vi "运维调试_总磷总氮.vi"() -> ()   [LabVIEW 2016, in "斯坦道氨氮.lvlib"]
uses:
  <vilib>/Utility/miscctls.llb/LVStringsAndValuesArrayTypeDef_U16.ctl
  <vilib>/Utility/miscctls.llb/LVPointTypeDef.ctl
  <vilib>/Plasmionique/MB Master/MB_Master/MB_Master.lvclass
  <vilib>/Utility/config.llb/NI_LVConfig.lvlib
  <vilib>/ptbypt/NI_PtbyPt.lvlib
panel:
  in  "灯值调整":bool
  in  "测试量程配置":T1
  in  "启动参数设置":bool
  out "固件版本号":string
  in  "定时设置":cluster{"启动":bool, "控制命令":T2, "测量参数":T3}(xcontrol)
  out "模块版本号":string
  out "温度2":sgl
  out "温度1":sgl
  out "ADC":sgl
  out "F3":sgl format="%#.6f"
  out "F2":sgl format="%#.6f"
  out "F1":sgl format="%#.6f"
  out "F0":sgl format="%#.6f"
  out "运行状态":T4 {"数据时间:" format="%<%y/%m/%d %H:%M:%S>T"; "仪器时间:" format="%<%y/%m/%d %H:%M:%S>T"}
  in  "单选按钮":enum32{"COD", "NH3N", "TN", "TP"}(radio)=enum."TN"
  in  "仪器参数":bool
  out "二级权限":bool
  out "一级权限":bool
  out "输入密码":u32
  out "布尔":bool
  in  "流程固件":bool
  in  "量程参数读取":T5
  in  "模块启用":bool
  in  "串口设置":bool
  in  "公式一键写入":bool
  in  "流程路径":path=path "data/流程.xml"
  in  "曲线模型":cluster{"X^2":dbl, "X":dbl, "B":dbl, "r^2":dbl}(xcontrol)
  out "字符串 2":string
  in  "质控参数设置":bool
  in  "数组":string[](array[string])
  in  "量程切换阈值写入":bool
  in  "量程切换阈值读取":bool
  in  "参数下拉列表":enum16{"COD", "氨氮", "总氮", "总磷"}(ring)
  in  "量程下拉列表":enum16{"低量程", "高量程"}(ring)
  in  "测量模式下拉列表":enum16{"水样测量", "零点核查", "跨度核查", "标样核查", "加标回收"}(ring)
  in  "公式":cluster{"X^2":dbl, "X":dbl, "b":dbl}
  in  "写公式":bool
  in  "读公式":bool
  in  "返回":bool
  in  "参数设置":bool
  out "集成报警信息":string
  in  "停止":bool
  in  "手动启动":bool
  in  "单步测试":bool
  out "多列列表框":i32(listbox)
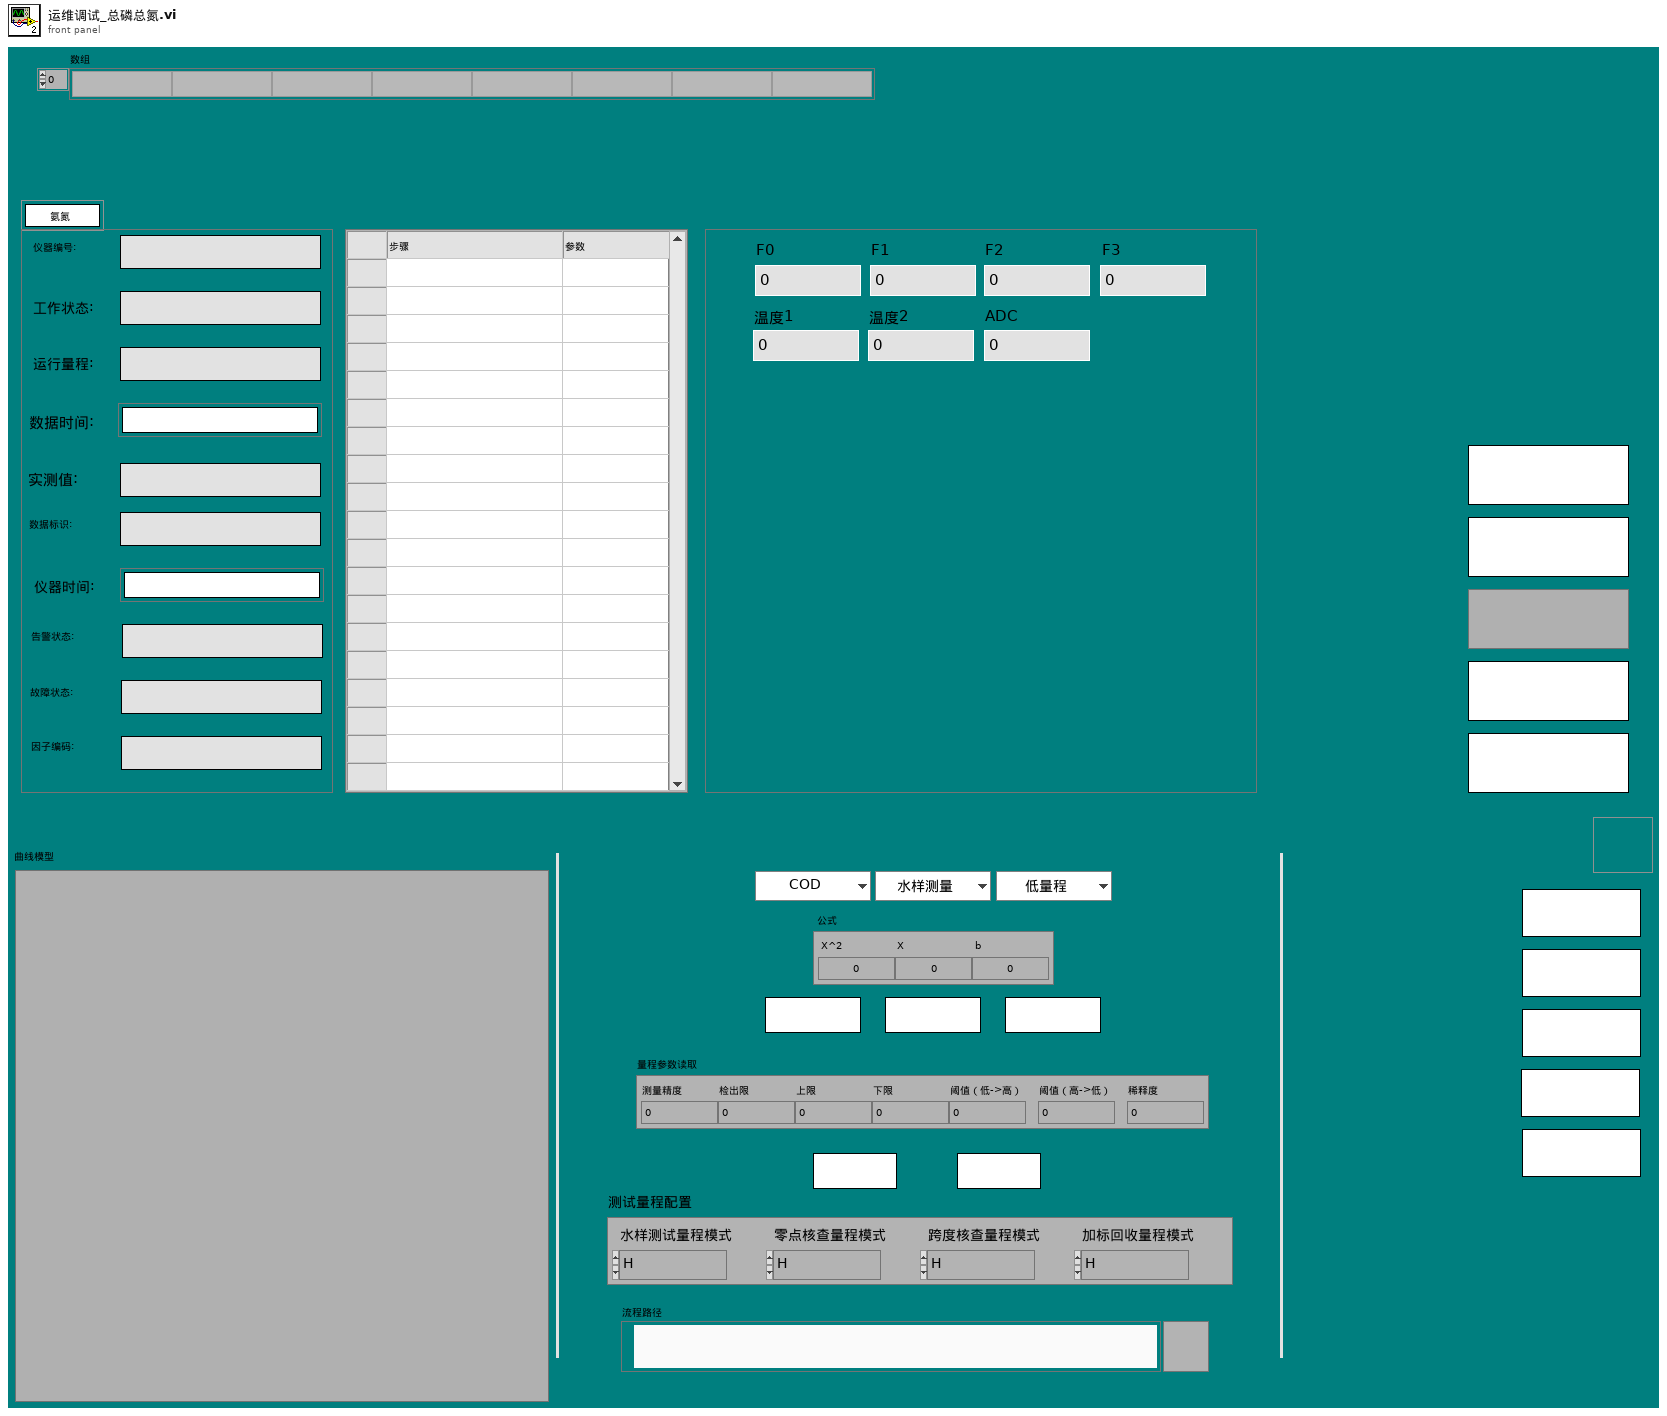
[diagram p1: front panel]
types:
  T1 = cluster{"水样测试量程模式":enum16{"H", "L", "AUTO"}, "空白核查量程模式":enum16{"H", "L", "AUTO"}, "跨度核查量程模式":enum16{"H", "L", "AUTO"}, "跨度核查量程模式 2":enum16{"H", "L", "AUTO"}}
  T2 = typedef "定时设置.xctl/国标控制命令.ctl" = enum16{"启动测量", "标样核查", "零点核查", "跨度核查", "空白测试", "平行样测试", "加标回收", "空白校准", "标样校准", "初始化（清洗）", "停止测试", "仪器重启", "校时", "模式设置", "测量间隔设置"}
  T3 = typedef "定时设置.xctl/测量参数.ctl" = u16
  T4 = cluster{"仪器编号:":string, "工作状态:":string, "运行量程: ":string, "数据时间:":timestamp, "实测值:":string, "数据标识: ":string, "仪器时间:":timestamp, "告警状态: ":string, "故障状态:  ":string, "因子编码:":string}
  T5 = cluster{"测量精度":dbl, "检出限":dbl, "上限":dbl, "下限":dbl, "阈值（低->高）":dbl, "阈值（高->低）":dbl, "稀释度":dbl}
  T6 = cluster{"时间源选择":enum16{"系统时间源", "仪器时间源"}, "外部时间源":timestamp}
  T7 = cluster{"系统时间":timestamp, "工作状态":enum16{"空闲", "水样测试", "标样核查", "零点核查", "跨度核查", "空白测试", "平行样测试", "加标回收", "空白校准", "标样校准", "初始化（清洗）"}, "测量模式":enum16{"待机", "连续模式", "周期模式", "定点模式", "受控模式", "手动模式"}, "告警代码":u16, "故障代码":u16, "日志代码":u16, "软件版本":u16, "F0":sgl, "F1":sgl, "F2":sgl, "F3":sgl, "T":sgl, "H":sgl, "id":u16, "flowid":u16, "量程":u16, "总磷控温温度1":sgl, "营养盐控温温度2":sgl, "ADC":sgl}
  T8 = enum32{"Bad", "Idle", "Run top level", "Running"}
  T9 = enum16{"空闲", "水样测试", "标样核查", "零点核查", "跨度核查", "空白测试", "平行样测试", "加标回收", "空白校准", "标样校准", "初始化（清洗）"}
  T10 = cluster{"水样测试量程模式":enum16{"H", "L", "AUTO"}, "空白核查量程模式":enum16{"H", "L", "AUTO"}, "跨度核查量程模式":enum16{"H", "L", "AUTO"}, "加标回收量程模式":enum16{"H", "L", "AUTO"}}
  T11 = typedef "LVStringsAndValuesArrayTypeDef_U16.ctl" = cluster{"String":string, "Value":u16}[]
  T12 = cluster{"COD":bool, "氨氮":bool, "总氮":bool, "总磷":bool}
  T13 = typedef "LVPointTypeDef.ctl" = cluster{"Horizontal":i16, "Vertical":i16}
  T14 = cluster{"因子编码":u32, "单位":u16, "标样参考值":sgl, "水样数据时间":timestamp, "水样实测值":sgl, "水样数据标识":string, "标样数据时间":timestamp, "标样实测值":sgl, "标样数据标识":string, "空白数据时间":timestamp, "空白实测值":sgl, "空白数据标识":string, "零点核查数据时间":timestamp, "零点核查实测值":sgl, "零点核查数据标识":string, "跨度核查数据时间":timestamp, "跨度核查实测值":sgl, "跨度核查数据标识":string, "加标回收数据时间":timestamp, "加标回收实测值":sgl, "加标回收数据标识":string, "平行样数据时间":timestamp, "平行样实测值":sgl, "平行样数据标识":string, "F0":sgl, "F1":sgl, "F2":sgl, "F3":sgl, "F4":sgl, "F5":sgl, "F6":sgl, "F7":sgl, "温度":sgl, "湿度":sgl, "X值":sgl, "fidrange":u16}
  T15 = cluster{"时间标识":timestamp, "设备":string, "日志信息":string, "备注":string}
  T16 = cluster{"参数":string, "报警内容":string, "报警分析":string}
  T17 = typedef "NI_LVConfig.lvlib/Config Data RefNum.ctl" = refnum<k1>
  T18 = cluster{"启动模式":enum16{"跨度核查", "水样测量", "空白核查", "标样核查", "加标回收"}, "启动参数":u16, "量程":enum16{"低量程", "高量程"}}
  T19 = cluster{"时间标识":timestamp, "设备":string, "日志信息":string, "流程参数":string}
  T20 = typedef "LVRowAndColumnUnsignedTypeDef.ctl" = cluster{"Row":u32, "Column":u32}
  T21 = cluster{"Major":u16, "Minor":u16, "Fix":u16, "Build":u16}
  T22 = cluster{"站号":u16, "量程切换":enum32{"H", "L", "AUTO"}, "控制命令":enum16{"启动测量", "标样核查", "零点核查", "跨度核查", "空白测试", "平行样测试", "加标回收", "空白校准", "标样校准", "初始化（清洗）", "停止测试", "仪器重启", "校时", "模式设置", "测量间隔设置"}, "模式设置":enum16{"待机", "连续模式", "周期模式", "定点模式", "受控模式", "手动模式"}, "测量间隔":u16}
  T23 = cluster{"参数下拉列表":enum16{"COD", "氨氮", "总氮", "总磷"}, "测量模式下拉列表":enum16{"水样测量", "零点核查", "跨度核查", "标样核查", "加标回收"}, "量程下拉列表":enum16{"低量程", "高量程"}}
  T24 = cluster{"被复制模型":cluster{"参数":u8, "测量模式":u8, "量程":u8}, "被覆盖模型":cluster{"参数":u8, "测量模式":u8, "量程":u8}[]}
  T25 = cluster{"总磷跨度值":dbl, "总磷零点标准液浓度":dbl, "总磷跨度标准液浓度":dbl, "总磷标准液标准浓度":dbl, "总氮跨度值":dbl, "总氮零点标准液浓度":dbl, "总氮跨度标准液浓度":dbl, "总氮标准液标准浓度":dbl, "COD跨度值":dbl, "COD零点标准液浓度":dbl, "COD跨度标准液浓度":dbl, "COD标准液标准浓度":dbl, "氨氮跨度值":dbl, "氨氮零点标准液浓度":dbl, "氨氮跨度标准液浓度":dbl, "氨氮标准液标准浓度":dbl}
  T26 = cluster{"测量量程":dbl, "测量精度":dbl, "测量间隔":dbl, "消解温度":dbl, "消解时长":dbl, "空白校准时间":timestamp, "曲线截距":dbl, "曲线斜率":dbl, "测量检出限":dbl, "测量信号值":dbl, "线性相关系数":dbl, "二次多项式系数":dbl, "标样校准时间":timestamp, "稀释倍数":dbl, "三项式系数":dbl, "空白标定系数":dbl, "量程系数":dbl, "F0/ORPA":dbl, "F1/ORPB":dbl, "F2/ORPK":dbl, "F3":dbl, "F4":dbl, "F5":dbl, "F6":dbl, "F7":dbl, "X0/滴定数":dbl, "量程":dbl}
  T27 = cluster{"COD仪器参数":cluster{"测量量程":dbl, "测量精度":dbl, "测量间隔":dbl, "消解温度":dbl, "消解时长":dbl, "空白校准时间":timestamp, "曲线截距":dbl, "曲线斜率":dbl, "测量检出限":dbl, "测量信号值":dbl, "线性相关系数":dbl, "二次多项式系数":dbl, "标样校准时间":timestamp, "稀释倍数":dbl, "三项式系数":dbl, "空白标定系数":dbl, "量程系数":dbl, "F0/ORPA":dbl, "F1/ORPB":dbl, "F2/ORPK":dbl, "F3":dbl, "F4":dbl, "F5":dbl, "F6":dbl, "F7":dbl, "X0/滴定数":dbl, "量程":dbl}, "氨氮仪器参数":cluster{"测量量程":dbl, "测量精度":dbl, "测量间隔":dbl, "消解温度":dbl, "消解时长":dbl, "空白校准时间":timestamp, "曲线截距":dbl, "曲线斜率":dbl, "测量检出限":dbl, "测量信号值":dbl, "线性相关系数":dbl, "二次多项式系数":dbl, "标样校准时间":timestamp, "稀释倍数":dbl, "三项式系数":dbl, "空白标定系数":dbl, "量程系数":dbl, "F0/ORPA":dbl, "F1/ORPB":dbl, "F2/ORPK":dbl, "F3":dbl, "F4":dbl, "F5":dbl, "F6":dbl, "F7":dbl, "X0/滴定数":dbl, "量程":dbl}, "总氮仪器参数":cluster{"测量量程":dbl, "测量精度":dbl, "测量间隔":dbl, "消解温度":dbl, "消解时长":dbl, "空白校准时间":timestamp, "曲线截距":dbl, "曲线斜率":dbl, "测量检出限":dbl, "测量信号值":dbl, "线性相关系数":dbl, "二次多项式系数":dbl, "标样校准时间":timestamp, "稀释倍数":dbl, "三项式系数":dbl, "空白标定系数":dbl, "量程系数":dbl, "F0/ORPA":dbl, "F1/ORPB":dbl, "F2/ORPK":dbl, "F3":dbl, "F4":dbl, "F5":dbl, "F6":dbl, "F7":dbl, "X0/滴定数":dbl, "量程":dbl}, "总磷仪器参数":cluster{"测量量程":dbl, "测量精度":dbl, "测量间隔":dbl, "消解温度":dbl, "消解时长":dbl, "空白校准时间":timestamp, "曲线截距":dbl, "曲线斜率":dbl, "测量检出限":dbl, "测量信号值":dbl, "线性相关系数":dbl, "二次多项式系数":dbl, "标样校准时间":timestamp, "稀释倍数":dbl, "三项式系数":dbl, "空白标定系数":dbl, "量程系数":dbl, "F0/ORPA":dbl, "F1/ORPB":dbl, "F2/ORPK":dbl, "F3":dbl, "F4":dbl, "F5":dbl, "F6":dbl, "F7":dbl, "X0/滴定数":dbl, "量程":dbl}}
  T28 = cluster{"测量精度":u16, "检出限":dbl, "上限":dbl, "下限":dbl, "阈值（低->高）":dbl, "阈值（高->低）":dbl, "稀释度":dbl}
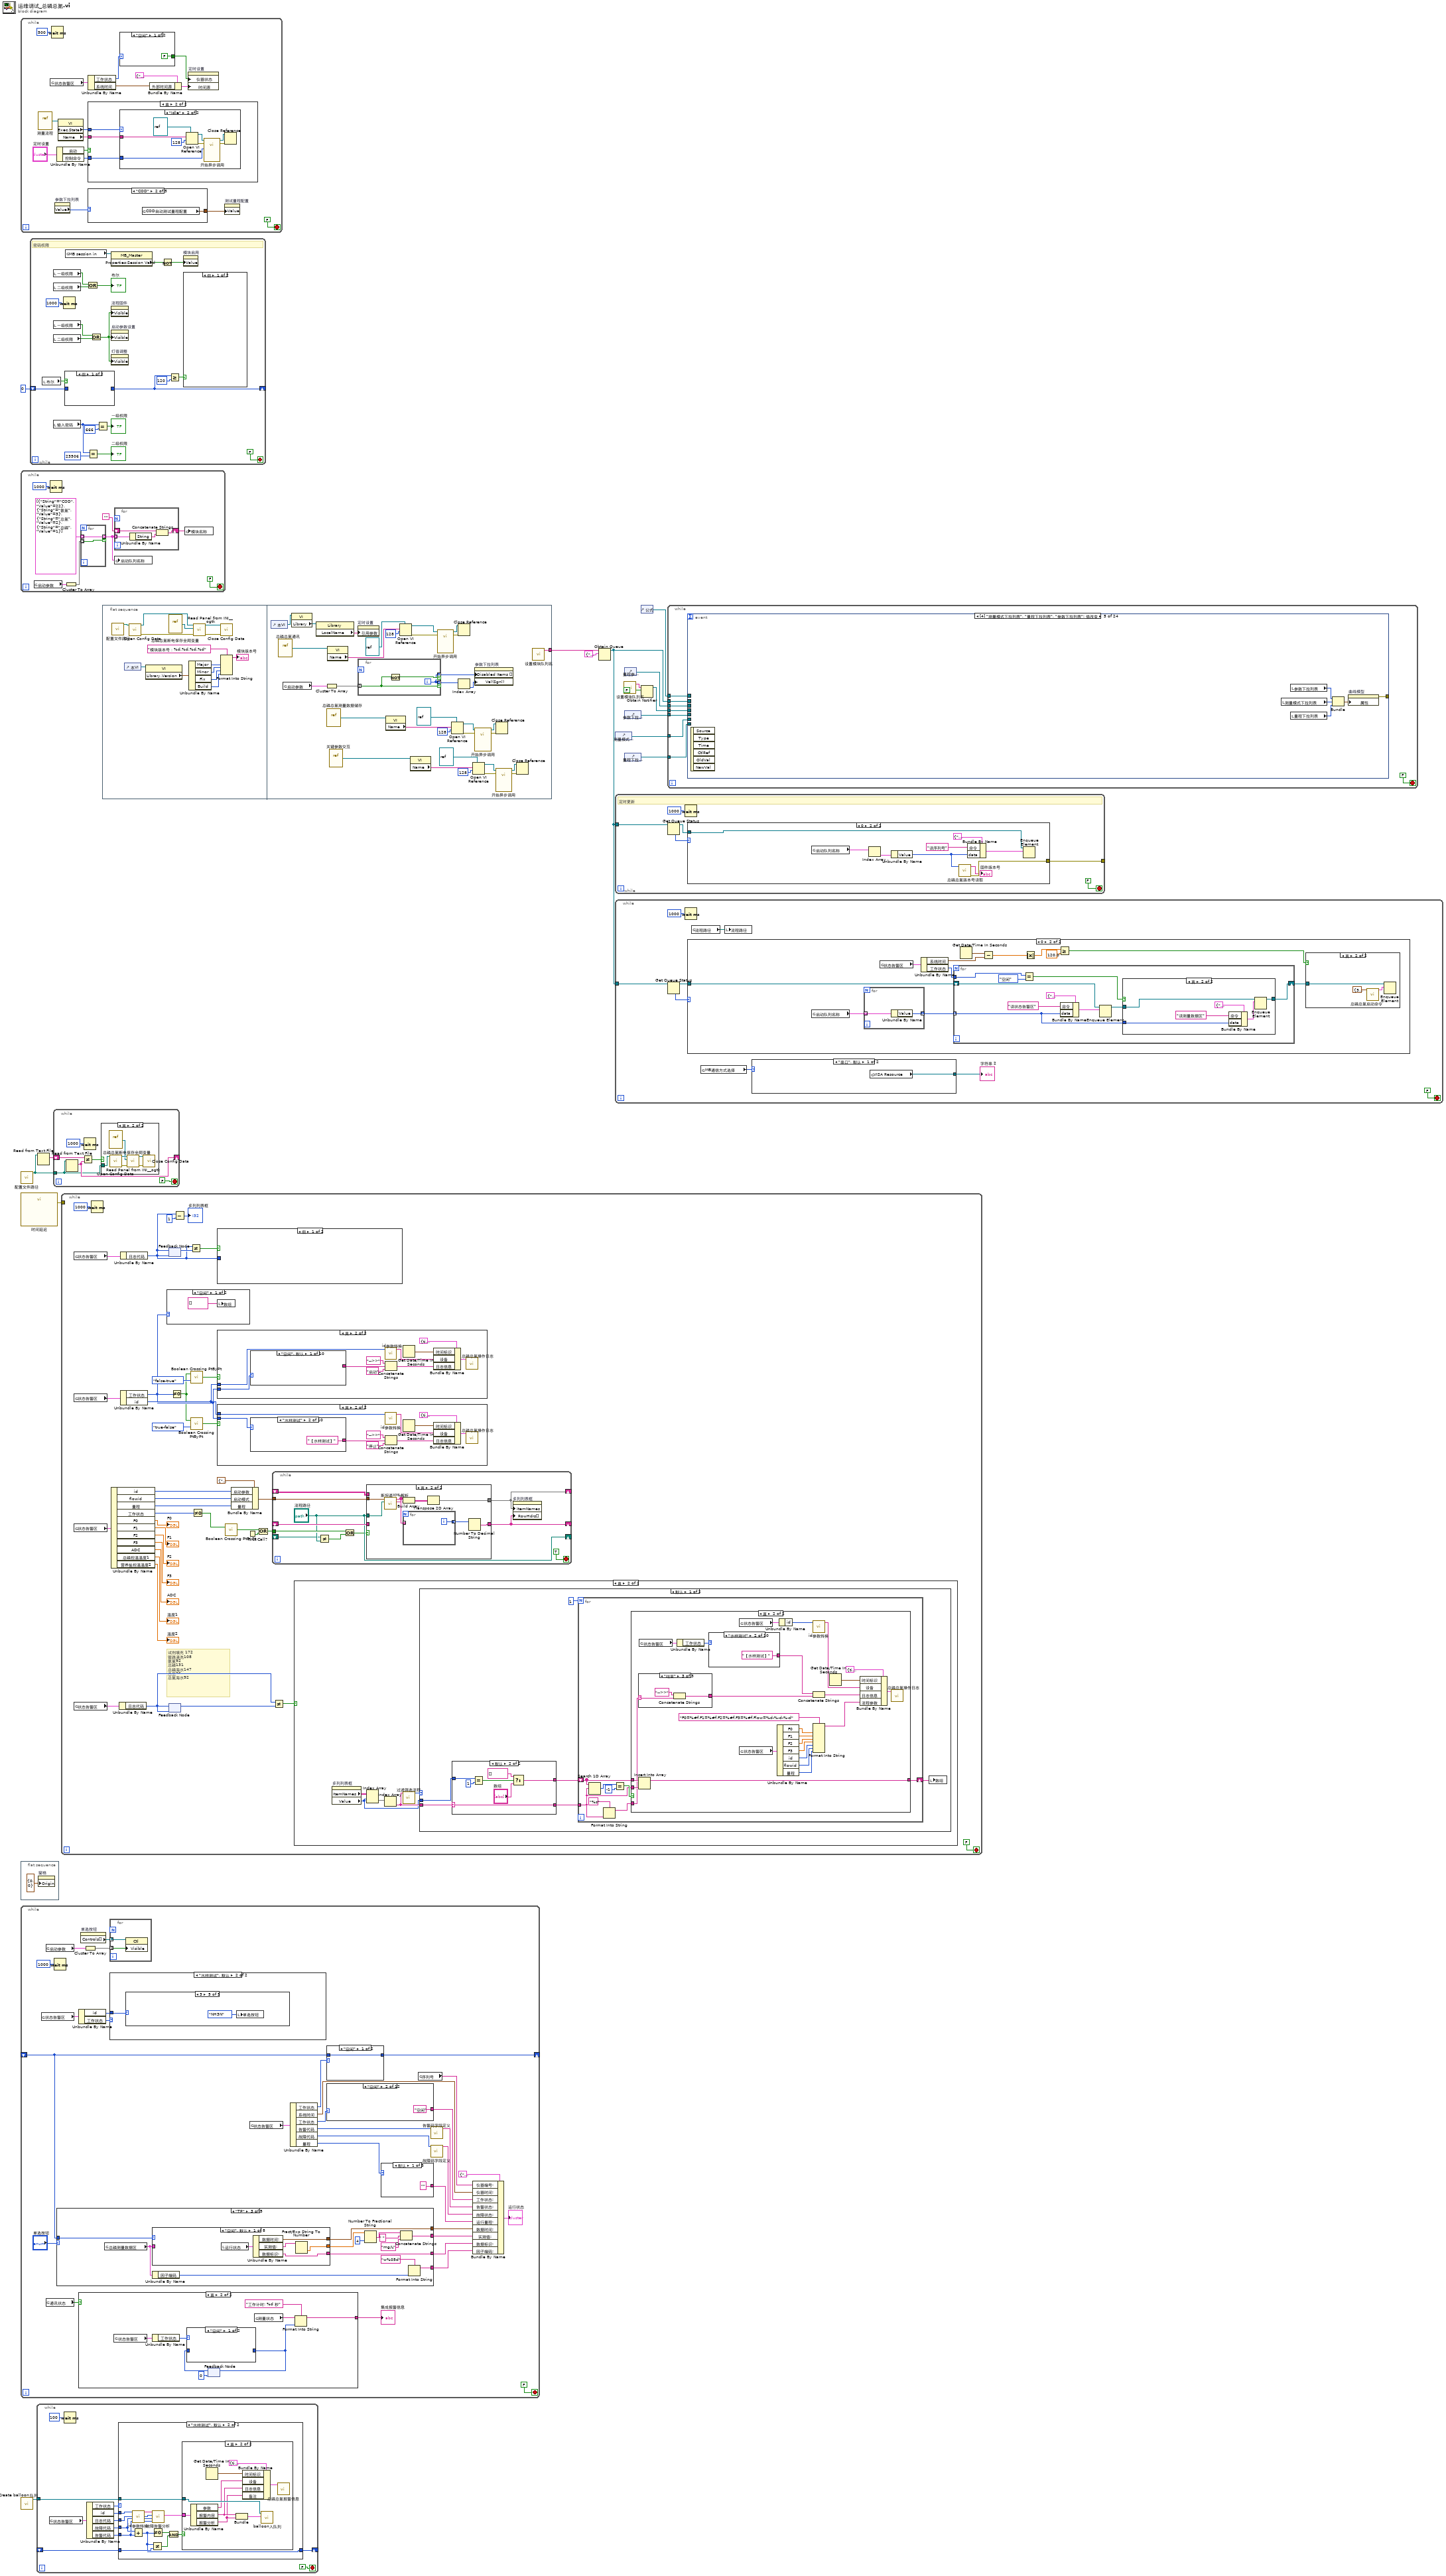
[diagram p0: block diagram]
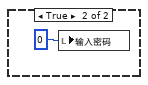
[diagram p5: hidden frame]
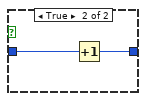
[diagram p6: hidden frame]
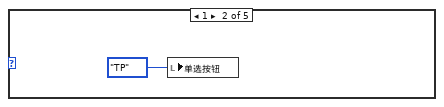
[diagram p11: hidden frame]
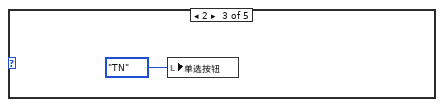
[diagram p12: hidden frame]
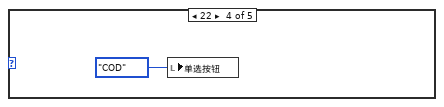
[diagram p13: hidden frame]
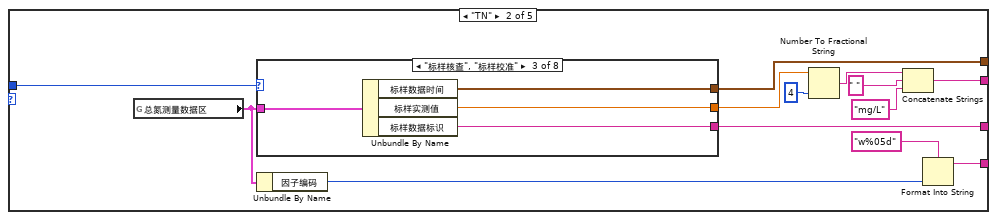
[diagram p15: hidden frame]
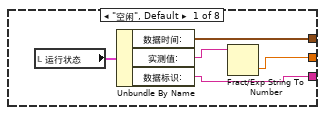
[diagram p16: hidden frame]
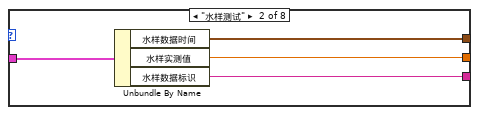
[diagram p17: hidden frame]
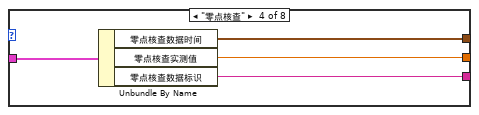
[diagram p18: hidden frame]
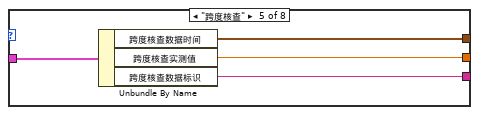
[diagram p19: hidden frame]
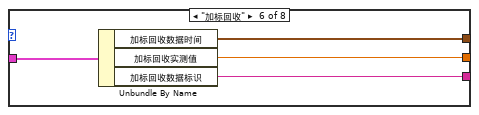
[diagram p20: hidden frame]
diagram:
  n1 = while {
    stop <- FALSE stop-if-true
    n2 = vi-ref "测量流程.vi"() -> (w30:refnum<vi>)
    n3 = global read "VAR总磷总氮全局变量.vi" "状态告警区"() -> (w27:T7)
    n4 = Wait (ms)(milliseconds to wait=u32 500 ("等待时间（毫秒）")) -> ()  [unwired: 1 out]
    n5 = property on="参数下拉列表" class="Enum (严格)"() -> ("Value"=w19:enum16{"COD", "氨氮", "总氮", "总磷"})  [unwired: 2 in, 2 out]
    n6 = Unbundle By Name("定时设置") -> ("启动"=w24:bool, "控制命令"=w23:T2)
    n7 = property class="VI"(reference=w30) -> ("Exec.State"=w29:T8, "Name"=w28:string)  [unwired: 1 in, 2 out]
    n8 = Unbundle By Name(w27) -> ("工作状态"=w26:T9, "系统时间"=w21:timestamp)
    n9 = case shown="真" w24 {
      tunnel: w28 -> [_ w41]
      tunnel: w23 -> [_ w40]
      tunnel: w29 -> [_ w39]
      frame False {
      }
      frame True {
        n10 = case shown="\"Idle\"" w39 {
          tunnel: w41 -> [_ w45]
          tunnel: w40 -> [_ w42]
          frame "Bad", Default {
          }
          frame "Idle" {
            n11 = Open VI Reference(type specifier VI Refnum (for type only)=refnum<vi> refnum, vi path=w45, options=128 ("选项")) -> (vi reference=w46:refnum<vi>, error out=w47:errorcluster)  [unwired: 3 in]
            n12 = call-by-ref "开始异步调用"(reference=w46, error in=w47, "控制命令"=w42) -> (reference out=w48:refnum<vi>, error out=w49:errorcluster)  [unwired: 11 in]
            n13 = Close Reference(reference=w48, error in (no error)=w49) -> ()  [unwired: 1 out]
          }
        }
      }
    }
    n14 = case shown="\"COD\"" w19 {
      tunnel: [_ w33 w34 w35 w36] -> w18
      frame Default {
      }
      frame "COD" {
        n15 = global read "总磷总氮断电保存全局变量.vi" "COD自动测试量程配置"() -> (w33:T10)
      }
      frame "氨氮" {
        n16 = global read "总磷总氮断电保存全局变量.vi" "氨氮自动测试量程配置"() -> (w34:T10)
      }
      frame "总氮" {
        n17 = global read "总磷总氮断电保存全局变量.vi" "总氮自动测试量程配置"() -> (w35:T10)
      }
      frame "总磷" {
        n18 = global read "总磷总氮断电保存全局变量.vi" "总磷自动测试量程配置"() -> (w36:T10)
      }
    }
    n19 = case shown="\"空闲\"" w26 {
      tunnel: [FALSE TRUE] -> w17
      frame "空闲" {
      }
      frame "水样测试", Default {
      }
    }
    n20 = Bundle By Name(cluster=T6 {"时间源选择"=enum."仪器时间源", "外部时间源"=timestamp(0 s since 1904-01-01)} ("时间源"), "外部时间源"=w21) -> (w20:T6)
    n21 = property on="定时设置" class="定时设置 (严格)"("仪器状态"=w17, "时间源"=w20) -> ()  [unwired: 2 in, 2 out]
    n22 = property on="测试量程配置" class="Clust (严格)"("Value"=w18) -> ()  [unwired: 2 in, 2 out]
  }
  n23 = while {
    stop <- FALSE stop-if-true
    n24 = global read "总磷总氮断电保存全局变量.vi" "启动参数"() -> (w55:T12)
    n25 = Wait (ms)(milliseconds to wait=u32 1000 ("等待时间（毫秒）")) -> ()  [unwired: 1 out]
    n26 = Cluster To Array(cluster=w55) -> (array=w54:bool[])
    n27 = for {
      tunnel: w54 -> [w63] mode=indexing
      tunnel: T11 [{"String"="COD", "Value"=22}, {"String"="氨氮", "Value"=3}, {"String"="总氮", "Value"=2}, {"String"="总磷", "Value"=1}] ("字符串与值[]") -> [w62] mode=indexing
      tunnel: [w62] -> w52 mode=indexing if=w63
    }
    n28 = for {
      tunnel: w52 -> [w61] mode=indexing
      shift-right: [w60] -> w50
      shift-left: "" -> [w58]
      n29 = Unbundle By Name(w61) -> ("String"=w59:string)
      n30 = Concatenate Strings(w58, w59) -> (w60:string)
    }
    n31 = global write "VAR总磷总氮全局变量.vi" "启动队列名称"(w52) -> ()
    n32 = global write "VAR总磷总氮全局变量.vi" "模块名称"(w50) -> ()
  }
  n33 = call "配置文件路径.vi"() -> ("appended path"=w4:path)  [unwired: 11 in]
  n34 = call "时间延迟"() -> ("error out"=w11:errorcluster)  [unwired: 11 in]
  n35 = flat-sequence {
    frame #0 {
      n36 = property on="窗格" class="Pane"("Origin"=T13 {"Horizontal"=0, "Vertical"=0} ("原点")) -> ()  [unwired: 2 in, 2 out]
    }
  }
  n37 = while {
    shift-right: [w66] -> _
    shift-left: _ -> [w65]
    stop <- FALSE stop-if-true
    n38 = global read "VAR总磷总氮全局变量.vi" "状态告警区"() -> (w77:T7)
    n39 = global read "总磷总氮断电保存全局变量.vi" "启动参数"() -> (w69:T12)
    n40 = global read "VAR总磷总氮全局变量.vi" "通讯状态"() -> (w93:bool)
    n41 = Wait (ms)(milliseconds to wait=u32 1000 ("等待时间（毫秒）")) -> ()  [unwired: 1 out]
    n42 = case shown="\"TP\"" "单选按钮" {
      tunnel: w65 -> [_ w109 w155 w201 w247]
      tunnel: [_ w108 w154 w199 w245] -> w81
      tunnel: [_ w107 w157 w203 w249] -> w80
      tunnel: [_ w106 w152 w197 w243] -> w79
      tunnel: [_ w105 w156 w202 w248] -> w78
      frame Default {
      }
      frame "TN" {
        n43 = global read "VAR总磷总氮全局变量.vi" "总氮测量数据区"() -> (w110:T14)
        n44 = case shown="\"标样核查\", \"标样校准\"" w109 {
          tunnel: [w120 w126 w130 w134 w138 w142 w146 w150] -> w108
          tunnel: [w118 w125 w129 w133 w136 w141 w145 w149] -> w112
          tunnel: [w121 w124 w128 w132 w135 w140 w144 w148] -> w106
          tunnel: w110 -> [_ w123 w127 w131 w137 w139 w143 w147]
          frame "空闲", Default {
            n45 = local read "运行状态"() -> (w122:T4)
            n46 = Unbundle By Name(w122) -> ("数据时间:"=w120:timestamp, "实测值:"=w119:string, "数据标识:"=w121:string)
            n47 = Fract/Exp String To Number(string=w119) -> (number=w118:dbl)  [unwired: 3 in, 1 out]
          }
          frame "水样测试" {
            n48 = Unbundle By Name(w123) -> ("水样数据时间"=w126:timestamp, "水样实测值"=w125:sgl, "水样数据标识"=w124:string)
          }
          frame "标样核查", "标样校准" {
            n49 = Unbundle By Name(w127) -> ("标样数据时间"=w130:timestamp, "标样实测值"=w129:sgl, "标样数据标识"=w128:string)
          }
          frame "零点核查" {
            n50 = Unbundle By Name(w131) -> ("零点核查数据时间"=w134:timestamp, "零点核查实测值"=w133:sgl, "零点核查数据标识"=w132:string)
          }
          frame "跨度核查" {
            n51 = Unbundle By Name(w137) -> ("跨度核查数据时间"=w138:timestamp, "跨度核查实测值"=w136:sgl, "跨度核查数据标识"=w135:string)
          }
          frame "加标回收" {
            n52 = Unbundle By Name(w139) -> ("加标回收数据时间"=w142:timestamp, "加标回收实测值"=w141:sgl, "加标回收数据标识"=w140:string)
          }
          frame "空白测试", "空白校准" {
            n53 = Unbundle By Name(w143) -> ("空白数据时间"=w146:timestamp, "空白实测值"=w145:sgl, "空白数据标识"=w144:string)
          }
          frame "平行样测试" {
            n54 = Unbundle By Name(w147) -> ("平行样数据时间"=w150:timestamp, "平行样实测值"=w149:sgl, "平行样数据标识"=w148:string)
          }
        }
        n55 = Unbundle By Name(w110) -> ("因子编码"=w116:u32)
        n56 = Number To Fractional String(number=w112, precision (6)=i16 4 ("精度(6)")) -> (F-format string=w114:string)  [unwired: 2 in]
        n57 = Concatenate Strings(w114, " " ("字符串"), "mg/L" ("字符串")) -> (w107:string)
        n58 = Format Into String(format string="w%05d" ("格式字符串"), w116) -> (resulting string=w105:string)  [unwired: 2 in, 1 out]
      }
      frame "TP" {
        n59 = global read "VAR总磷总氮全局变量.vi" "总磷测量数据区"() -> (w151:T14)
        n60 = case shown="\"空闲\", 默认" w155 {
          tunnel: [w166 w172 w176 w180 w184 w188 w192 w196] -> w154
          tunnel: [w164 w171 w175 w179 w182 w187 w191 w195] -> w153
          tunnel: [w167 w170 w174 w178 w181 w186 w190 w194] -> w152
          tunnel: w151 -> [_ w169 w173 w177 w183 w185 w189 w193]
          frame "空闲", Default {
            n61 = local read "运行状态"() -> (w168:T4)
            n62 = Unbundle By Name(w168) -> ("数据时间:"=w166:timestamp, "实测值:"=w165:string, "数据标识:"=w167:string)
            n63 = Fract/Exp String To Number(string=w165) -> (number=w164:dbl)  [unwired: 3 in, 1 out]
          }
          frame "水样测试" {
            n64 = Unbundle By Name(w169) -> ("水样数据时间"=w172:timestamp, "水样实测值"=w171:sgl, "水样数据标识"=w170:string)
          }
          frame "标样核查" {
            n65 = Unbundle By Name(w173) -> ("标样数据时间"=w176:timestamp, "标样实测值"=w175:sgl, "标样数据标识"=w174:string)
          }
          frame "零点核查" {
            n66 = Unbundle By Name(w177) -> ("零点核查数据时间"=w180:timestamp, "零点核查实测值"=w179:sgl, "零点核查数据标识"=w178:string)
          }
          frame "跨度核查" {
            n67 = Unbundle By Name(w183) -> ("跨度核查数据时间"=w184:timestamp, "跨度核查实测值"=w182:sgl, "跨度核查数据标识"=w181:string)
          }
          frame "加标回收" {
            n68 = Unbundle By Name(w185) -> ("加标回收数据时间"=w188:timestamp, "加标回收实测值"=w187:sgl, "加标回收数据标识"=w186:string)
          }
          frame "空白测试" {
            n69 = Unbundle By Name(w189) -> ("空白数据时间"=w192:timestamp, "空白实测值"=w191:sgl, "空白数据标识"=w190:string)
          }
          frame "平行样测试" {
            n70 = Unbundle By Name(w193) -> ("平行样数据时间"=w196:timestamp, "平行样实测值"=w195:sgl, "平行样数据标识"=w194:string)
          }
        }
        n71 = Unbundle By Name(w151) -> ("因子编码"=w162:u32)
        n72 = Number To Fractional String(number=w153, precision (6)=i16 4 ("精度(6)")) -> (F-format string=w160:string)  [unwired: 2 in]
        n73 = Concatenate Strings(w160, " " ("字符串"), "mg/L" ("字符串")) -> (w157:string)
        n74 = Format Into String(format string="w%05d" ("格式字符串"), w162) -> (resulting string=w156:string)  [unwired: 2 in, 1 out]
      }
      frame "NH3N" {
        n75 = global read "VAR总磷总氮全局变量.vi" "氨氮测量数据区"() -> (w200:T14)
        n76 = case shown="\"空闲\", 默认" w201 {
          tunnel: [w212 w218 w222 w226 w230 w234 w238 w242] -> w199
          tunnel: [w210 w217 w221 w225 w228 w233 w237 w241] -> w198
          tunnel: [w213 w216 w220 w224 w227 w232 w236 w240] -> w197
          tunnel: w200 -> [_ w215 w219 w223 w229 w231 w235 w239]
          frame "空闲", Default {
            n77 = local read "运行状态"() -> (w214:T4)
            n78 = Unbundle By Name(w214) -> ("数据时间:"=w212:timestamp, "实测值:"=w211:string, "数据标识:"=w213:string)
            n79 = Fract/Exp String To Number(string=w211) -> (number=w210:dbl)  [unwired: 3 in, 1 out]
          }
          frame "水样测试" {
            n80 = Unbundle By Name(w215) -> ("水样数据时间"=w218:timestamp, "水样实测值"=w217:sgl, "水样数据标识"=w216:string)
          }
          frame "标样核查" {
            n81 = Unbundle By Name(w219) -> ("标样数据时间"=w222:timestamp, "标样实测值"=w221:sgl, "标样数据标识"=w220:string)
          }
          frame "零点核查" {
            n82 = Unbundle By Name(w223) -> ("零点核查数据时间"=w226:timestamp, "零点核查实测值"=w225:sgl, "零点核查数据标识"=w224:string)
          }
          frame "跨度核查" {
            n83 = Unbundle By Name(w229) -> ("跨度核查数据时间"=w230:timestamp, "跨度核查实测值"=w228:sgl, "跨度核查数据标识"=w227:string)
          }
          frame "加标回收" {
            n84 = Unbundle By Name(w231) -> ("加标回收数据时间"=w234:timestamp, "加标回收实测值"=w233:sgl, "加标回收数据标识"=w232:string)
          }
          frame "空白测试" {
            n85 = Unbundle By Name(w235) -> ("空白数据时间"=w238:timestamp, "空白实测值"=w237:sgl, "空白数据标识"=w236:string)
          }
          frame "平行样测试" {
            n86 = Unbundle By Name(w239) -> ("平行样数据时间"=w242:timestamp, "平行样实测值"=w241:sgl, "平行样数据标识"=w240:string)
          }
        }
        n87 = Unbundle By Name(w200) -> ("因子编码"=w208:u32)
        n88 = Number To Fractional String(number=w198, precision (6)=i16 4 ("精度(6)")) -> (F-format string=w206:string)  [unwired: 2 in]
        n89 = Concatenate Strings(w206, " " ("字符串"), "mg/L" ("字符串")) -> (w203:string)
        n90 = Format Into String(format string="w%05d" ("格式字符串"), w208) -> (resulting string=w202:string)  [unwired: 2 in, 1 out]
      }
      frame "COD" {
        n91 = global read "VAR总磷总氮全局变量.vi" "COD测量数据区"() -> (w246:T14)
        n92 = case shown="\"空闲\", 默认" w247 {
          tunnel: [w258 w264 w268 w272 w276 w280 w284 w288] -> w245
          tunnel: [w256 w263 w267 w271 w274 w279 w283 w287] -> w244
          tunnel: [w259 w262 w266 w270 w273 w278 w282 w286] -> w243
          tunnel: w246 -> [_ w261 w265 w269 w275 w277 w281 w285]
          frame "空闲", Default {
            n93 = local read "运行状态"() -> (w260:T4)
            n94 = Unbundle By Name(w260) -> ("数据时间:"=w258:timestamp, "实测值:"=w257:string, "数据标识:"=w259:string)
            n95 = Fract/Exp String To Number(string=w257) -> (number=w256:dbl)  [unwired: 3 in, 1 out]
          }
          frame "水样测试" {
            n96 = Unbundle By Name(w261) -> ("水样数据时间"=w264:timestamp, "水样实测值"=w263:sgl, "水样数据标识"=w262:string)
          }
          frame "标样核查" {
            n97 = Unbundle By Name(w265) -> ("标样数据时间"=w268:timestamp, "标样实测值"=w267:sgl, "标样数据标识"=w266:string)
          }
          frame "零点核查" {
            n98 = Unbundle By Name(w269) -> ("零点核查数据时间"=w272:timestamp, "零点核查实测值"=w271:sgl, "零点核查数据标识"=w270:string)
          }
          frame "跨度核查" {
            n99 = Unbundle By Name(w275) -> ("跨度核查数据时间"=w276:timestamp, "跨度核查实测值"=w274:sgl, "跨度核查数据标识"=w273:string)
          }
          frame "加标回收" {
            n100 = Unbundle By Name(w277) -> ("加标回收数据时间"=w280:timestamp, "加标回收实测值"=w279:sgl, "加标回收数据标识"=w278:string)
          }
          frame "空白测试" {
            n101 = Unbundle By Name(w281) -> ("空白数据时间"=w284:timestamp, "空白实测值"=w283:sgl, "空白数据标识"=w282:string)
          }
          frame "平行样测试" {
            n102 = Unbundle By Name(w285) -> ("平行样数据时间"=w288:timestamp, "平行样实测值"=w287:sgl, "平行样数据标识"=w286:string)
          }
        }
        n103 = Unbundle By Name(w246) -> ("因子编码"=w254:u32)
        n104 = Number To Fractional String(number=w244, precision (6)=i16 4 ("精度(6)")) -> (F-format string=w252:string)  [unwired: 2 in]
        n105 = Concatenate Strings(w252, " " ("字符串"), "mg/L" ("字符串")) -> (w249:string)
        n106 = Format Into String(format string="w%05d" ("格式字符串"), w254) -> (resulting string=w248:string)  [unwired: 2 in, 1 out]
      }
    }
    n107 = Unbundle By Name(w77) -> ("id"=w76:u16, "工作状态"=w71:T9)
    n108 = case shown="真" w93 {
      tunnel: ["通讯异常" ("集成报警信息") w309] -> w92
      frame False {
      }
      frame True {
        n109 = global read "VAR总磷总氮全局变量.vi" "状态告警区"() -> (w315:T7)
        n110 = Unbundle By Name(w315) -> ("工作状态"=w314:T9)
        n111 = feedback #1(0) -> (w312:i32)
        n112 = case shown="\"空闲\"" w314 {
          tunnel: w312 -> [_ w317]
          tunnel: [_ w316] -> w310
          frame "空闲" {
          }
          frame Default {
            n113 = Increment(x=w317) -> (x+1=w316:i32)
          }
        }
        n114 = feedback-in #1(w310) -> ()
        n115 = global read "VAR总磷总氮全局变量.vi" "测量状态"() -> (w308:string)
        n116 = Format Into String(format string="工作计时: %d 秒" ("格式字符串"), initial string=w308, w310) -> (resulting string=w309:string)  [unwired: 1 in, 1 out]
      }
    }
    "集成报警信息" <- w92
    n117 = property on="单选按钮" class="RadioBtnsControl (严格)"() -> ("Controls[]"=w70:refnum<vi>[])  [unwired: 2 in, 2 out]
    n118 = Cluster To Array(cluster=w69) -> (array=w68:bool[])
    n119 = for {
      tunnel: w70 -> [w99] mode=indexing
      tunnel: w68 -> [w98] mode=indexing
      n120 = property class="Ctl"(reference=w99, "Visible"=w98) -> ()  [unwired: 1 in, 2 out]
    }
    n121 = case shown="\"水样测试\", 默认" w71 {
      tunnel: w76 -> [_ w100]
      frame "空闲" {
      }
      frame "水样测试", Default {
        n122 = case shown="3" w100 {
          frame 0, Default {
          }
          frame 1 {
            n123 = local write "单选按钮"(enum32{"COD", "NH3N", "TN", "TP"}."TP" ("单选按钮")) -> ()
          }
          frame 2 {
            n124 = local write "单选按钮"(enum32{"COD", "NH3N", "TN", "TP"}."TN" ("单选按钮")) -> ()
          }
          frame 22 {
            n125 = local write "单选按钮"(enum32{"COD", "NH3N", "TN", "TP"}."COD" ("单选按钮")) -> ()
          }
          frame 3 {
            n126 = local write "单选按钮"(enum32{"COD", "NH3N", "TN", "TP"}."NH3N" ("单选按钮")) -> ()
          }
        }
      }
    }
    n127 = global read "VAR总磷总氮全局变量.vi" "状态告警区"() -> (w91:T7)
    n128 = Unbundle By Name(w91) -> ("工作状态"=w67:T9, "系统时间"=w87:timestamp, "工作状态"=w86:T9, "告警代码"=w75:u16, "故障代码"=w73:u16, "量程"=w84:u16)
    n129 = case shown="\"空闲\"" w67 {
      selector: w67 -> [_ w97]
      tunnel: [w96 w97] -> w66
      tunnel: w65 -> [w96 _]
      frame "空闲" {
      }
      frame "水样测试", Default {
      }
    }
    n130 = case shown="\"空闲\"" w86 {
      selector: w86 -> [w292 _ _ _ _ _ _ _ _ _ _ _]
      tunnel: [w293 "空闲" ("工作状态") "水样测量" ("工作状态") "标样核查" ("工作状态") "零点核查" ("工作状态") "跨度核查" ("工作状态") "空白测试" ("工作状态") "平行样测试" ("工作状态") "加标回收" ("工作状态") "空白校准" ("工作状态") "标样校准" ("工作状态") "初始化" ("工作状态")] -> w85
      frame Default {
        n131 = Format Into String(format string="%d" ("格式字符串"), initial string="未知" ("工作状态"), w292) -> (resulting string=w293:string)  [unwired: 1 in, 1 out]
      }
      frame "空闲" {
      }
      frame "水样测试" {
      }
      frame "标样核查" {
      }
      frame "零点核查" {
      }
      frame "跨度核查" {
      }
      frame "空白测试" {
      }
      frame "平行样测试" {
      }
      frame "加标回收" {
      }
      frame "空白校准" {
      }
      frame "标样校准" {
      }
      frame "初始化（清洗）" {
      }
    }
    n132 = case shown="默认" w84 {
      tunnel: ["" ("字符串") "低量程" ("字符串") "高量程" ("字符串")] -> w83
      frame Default {
      }
      frame 0 {
      }
      frame 1 {
      }
    }
    n133 = global read "VAR总磷总氮全局变量.vi" "序列号"() -> (w88:string)
    n134 = call "告警码字段定义.vi"("告警代码"=w75) -> ("字符串"=w74:string)  [unwired: 8 in, 2 out]
    n135 = call "故障码字段定义.vi"("故障代码"=w73) -> ("字符串"=w72:string)  [unwired: 10 in]
    n136 = Bundle By Name(cluster=T4 {"仪器编号:"="", "工作状态:"="", "运行量程: "="", "数据时间:"=timestamp(0 s since 1904-01-01), "实测值:"="", "数据标识: "="", "仪器时间:"=timestamp(0 s since 1904-01-01), "告警状态: "="", "故障状态:  "="", "因子编码:"=""} ("运行状态"), "仪器编号:"=w88, "仪器时间:"=w87, "工作状态:"=w85, "告警状态:"=w74, "故障状态:"=w72, "运行量程:"=w83, "数据时间:"=w81, "实测值:"=w80, "数据标识:"=w79, "因子编码:"=w78) -> (→"运行状态":T4)
  }
  n137 = call "Create balloon 队列.vi"() -> ("队列输出"=w8:refnum<queue>)  [unwired: 11 in]
  n138 = while {
    shift-right: [w326] -> _
    shift-left: u32 0 ("y") -> [w328]
    stop <- FALSE stop-if-true
    # "密码权限"
    n139 = local read "布尔"() -> (w329:bool)
    n140 = local read "一级权限"() -> (w331:bool)
    n141 = local read "二级权限"() -> (w332:bool)
    n142 = local read "一级权限"() -> (w322:bool)
    n143 = local read "二级权限"() -> (w323:bool)
    n144 = local read "输入密码"() -> (w335:u32)
    n145 = Wait (ms)(milliseconds to wait=u32 1000 ("等待时间（毫秒）")) -> ()  [unwired: 1 out]
    n146 = case shown="假" w329 {
      tunnel: w328 -> [_ w341]
      tunnel: [_ w340] -> w326
      frame False {
      }
      frame True {
        n147 = Increment(x=w341) -> (x+1=w340:u32)
      }
    }
    n148 = global read "VAR总磷总氮全局变量.vi" "MB session in"() -> (w321:refnum<class "MB_Master.lvclass">)
    n149 = Or(x=w331, y=w332) -> (x .or. y?=→"布尔":bool)
    n150 = Equal?(x=w335, y=u32 23506) -> (x = y?=→"二级权限":bool)
    n151 = Or(x=w322, y=w323) -> (x .or. y?=w318:bool)
    n152 = Equal?(x=w335, y=u32 666) -> (x = y?=→"一级权限":bool)
    n153 = property class="MB_Master"(reference=w321) -> ("Properties:Session Valid"=w320:bool)  [unwired: 1 in, 2 out]
    n154 = property on="流程固件" class="Bool"("Visible"=w318) -> ()  [unwired: 2 in, 2 out]
    n155 = property on="启动参数设置" class="Bool"("Visible"=w318) -> ()  [unwired: 2 in, 2 out]
    n156 = property on="灯值调整" class="Bool"("Visible"=w318) -> ()  [unwired: 2 in, 2 out]
    n157 = Not(x=w320) -> (.not. x?=w319:bool)
    n158 = Greater Or Equal?(x=w326, y=u32 120) -> (x >= y?=w324:bool)
    n159 = property on="模块启用" class="Bool (严格)"("Value"=w319) -> ()  [unwired: 2 in, 2 out]
    n160 = case shown="假" w324 {
      frame False {
      }
      frame True {
        n161 = local write "输入密码"(u32 0 ("输入密码")) -> ()
      }
    }
  }
  n162 = while {
    tunnel: w8 -> [w348]
    shift-right: [w344] -> _
    shift-left: _ -> [w345]
    stop <- FALSE stop-if-true
    n163 = global read "VAR总磷总氮全局变量.vi" "状态告警区"() -> (w342:T7)
    n164 = Wait (ms)(milliseconds to wait=u32 100) -> ()  [unwired: 1 out]
    n165 = Unbundle By Name(w342) -> ("工作状态"=w343:T9, "id"=w350:u16, "日志代码"=w349:u16, "故障代码"=w347:u16, "告警代码"=w346:u16)
    n166 = case shown="\"水样测试\", 默认" w343 {
      tunnel: w350 -> [_ w365]
      tunnel: w349 -> [_ w364]
      tunnel: w348 -> [_ w361]
      tunnel: w347 -> [_ w360]
      tunnel: w346 -> [_ w359]
      tunnel: w345 -> [w353 w358]
      tunnel: [w353 w357] -> w344
      frame "空闲" {
      }
      frame "水样测试", Default {
        n167 = call "id参数转换.vi"("id"=w365) -> ("table输出"=w362:string)  [unwired: 10 in]
        n168 = Add(x=w360, y=w359) -> (x+y=w357:u16)
        n169 = Not Equal?(x=w357, y=w358) -> (x != y?=w355:bool)
        n170 = Not Equal To 0?(x=w357) -> (x != 0?=w356:bool)
        n171 = call "故障告警分析.vi"("告警代码"=w359, "故障代码"=w360, "运行步序"=w364, "参数"=w362) -> ("报警内容"=w363:T16)  [unwired: 6 in, 1 out]
        n172 = And(x=w356, y=w355) -> (x .and. y?=w354:bool)
        n173 = case shown="真" w354 {
          tunnel: w363 -> [_ w374]
          tunnel: w361 -> [_ w373]
          frame False {
          }
          frame True {
            n174 = Unbundle By Name(w374) -> ("参数"=w369:string, "报警内容"=w368:string, "报警分析"=w367:string)
            n175 = Get Date/Time In Seconds() -> (seconds since 1Jan1904=w372:timestamp)
            n176 = Bundle("报警内容"=w368, "报警分析"=w367) -> (w366:cluster{"报警内容":string, "报警分析":string})  [unwired: 1 in]
            n177 = Bundle By Name(cluster=T15 {"时间标识"=timestamp(0 s since 1904-01-01), "设备"="", "日志信息"="", "备注"=""} ("data in"), "时间标识"=w372, "设备"=w369, "日志信息"=w368, "备注"=w367) -> (w371:T15)
            n178 = call "balloon入队列.vi"("报警内容"=w366, "队列"=w373) -> ()  [unwired: 9 in, 1 out]
            n179 = call "总磷总氮报警信息.vi"("data in"=w371) -> ()  [unwired: 10 in, 1 out]
          }
        }
      }
    }
  }
  n180 = Read from Text File(file (use dialog)=w4) -> (text=w5:string)  [unwired: 3 in, 3 out]
  n181 = while {
    shift-right: [w377] -> _
    shift-left: w5 -> [w379]
    tunnel: w4 -> [w376]
    stop <- FALSE stop-if-true
    n182 = Read from Text File(file (use dialog)=w376) -> (text=w377:string)  [unwired: 3 in, 3 out]
    n183 = Not Equal?(x=w379, y=w377) -> (x != y?=w378:bool)
    n184 = Wait (ms)(milliseconds to wait=u32 1000 ("等待时间（毫秒）")) -> ()  [unwired: 1 out]
    n185 = case shown="真" w378 {
      tunnel: w376 -> [_ w381]
      frame False {
      }
      frame True {
        n186 = vi-ref "总磷总氮断电保存全局变量.vi"() -> (w385:refnum<vi>)
        n187 = call <vilib>:"Open Config Data.vi"("configuration file path"=w381) -> ("error out"=w383:errorcluster, "refnum"=w386:T17)  [unwired: 8 in, 1 out]
        n188 = call <userlib>:"Read Panel from INI__ogtk.vi"("error in (no error)"=w383, "VI ref"=w385, "refnum"=w386) -> ("error out"=w382:errorcluster, "refnum out"=w384:T17)  [unwired: 7 in]
        n189 = call <vilib>:"Close Config Data.vi"("error in (no error)"=w382, "refnum"=w384) -> ()  [unwired: 8 in, 2 out]
      }
    }
  }
  n190 = while {
    tunnel: w11 -> [_]
    stop <- FALSE stop-if-true
    # "试剂填充 172 \n管路清洗108\n氨氮92\n总磷131\n总磷海水147\n总氮76\n总氮海水92"
    n191 = global read "VAR总磷总氮全局变量.vi" "状态告警区"() -> (w413:T7)
    n192 = global read "VAR总磷总氮全局变量.vi" "状态告警区"() -> (w411:T7)
    n193 = global read "VAR总磷总氮全局变量.vi" "状态告警区"() -> (w417:T7)
    n194 = global read "VAR总磷总氮全局变量.vi" "状态告警区"() -> (w409:T7)
    n195 = Wait (ms)(milliseconds to wait=u32 1000 ("等待时间（毫秒）")) -> ()  [unwired: 1 out]
    n196 = Unbundle By Name(w417) -> ("id"=w414:u16, "flowid"=w416:u16, "量程"=w415:u16, "工作状态"=w402:T9, "F0"=→"F0":sgl, "F1"=→"F1":sgl, "F2"=→"F2":sgl, "F3"=→"F3":sgl, "ADC"=→"ADC":sgl, "总磷控温温度1"=→"温度1":sgl, "营养盐控温温度2"=→"温度2":sgl)
    n197 = Unbundle By Name(w409) -> ("日志代码"=w408:u16)
    n198 = Unbundle By Name(w413) -> ("日志代码"=w405:u16)
    n199 = Unbundle By Name(w411) -> ("工作状态"=w397:T9, "id"=w398:u16)
    n200 = case shown="\"空闲\"" w397 {
      frame "空闲" {
        n201 = local write "数组"(string[] [] ("数组")) -> ()
      }
      frame "水样测试", Default {
      }
    }
    n202 = feedback-in #2(w405) -> ()
    n203 = feedback #2(w405) -> (w422:u16)
    n204 = feedback #3(w408) -> (w410:u16)
    n205 = feedback-in #3(w408) -> ()
    n206 = Not Equal To 0?(x=w397) -> (x != 0?=w395:bool)
    n207 = Subtract(x=w405, y=1) -> (x-y=→"多列列表框":i32)
    n208 = Not Equal?(x=w405, y=w422) -> (x != y?=w421:bool)
    n209 = call <vilib>:"Boolean Crossing PtByPt.vi"("direction"=enum16{"either", "false-true", "true-false"}."false-true", "input"=w395) -> ("crossing"=w399:bool)  [unwired: 1 in]
    n210 = call <vilib>:"Boolean Crossing PtByPt.vi"("direction"=enum16{"either", "false-true", "true-false"}."true-false", "input"=w395) -> ("crossing"=w394:bool)  [unwired: 1 in]
    n211 = Not Equal To 0?(x=w402) -> (x != 0?=w419:bool)
    n212 = case shown="假" w421 {
      tunnel: w405 -> [_ w558]
      frame False {
      }
      frame True {
        n213 = Subtract(x=w558, y=1) -> (x-y=w556:i32)
        n214 = Subtract(x=w556, y=5) -> (x-y=w560:i32)
        n215 = Greater Or Equal To 0?(x=w560) -> (x >= 0?=w559:bool)
        n216 = property on="多列列表框" class="MCListbox (严格)"() -> (error out=w564:errorcluster, "TopLeft"=w565:T20)  [unwired: 2 in, 1 out]
        n217 = Select(t=w560, s=w559, f=0) -> (s? t:f=w561:i32)
        n218 = Bundle By Name(cluster=w565, "Row"=w561) -> (w566:T20)
        n219 = property on="多列列表框" class="MCListbox (严格)"(error in=w564, "TopLeft"=w566) -> ()  [unwired: 1 in, 2 out]
      }
    }
    n220 = case shown="真" w399 {
      tunnel: w397 -> [_ w448]
      tunnel: w398 -> [_ w445]
      frame False {
      }
      frame True {
        n221 = case shown="\"空闲\", 默认" w448 {
          tunnel: [_ "【水样测试】" ("字符串") "【标样核查】" ("字符串") "【零点核查】" ("字符串") "【跨度核查】" ("字符串") "【空白测试】" ("字符串") "【平行样测试】" ("字符串") "【加标回收】" ("字符串") "【空白校准】" ("字符串") "【标样校准】" ("字符串")] -> w453
          frame "空闲", Default {
          }
          frame "水样测试" {
          }
          frame "标样核查" {
          }
          frame "零点核查" {
          }
          frame "跨度核查" {
          }
          frame "空白测试" {
          }
          frame "平行样测试" {
          }
          frame "加标回收" {
          }
          frame "空白校准" {
          }
          frame "标样校准" {
          }
        }
        n222 = call "id参数转换.vi"("id"=w445) -> ("table输出"=w444:string)  [unwired: 10 in]
        n223 = Concatenate Strings("-->>" ("字符串"), w453, "启动" ("字符串")) -> (w452:string)
        n224 = Get Date/Time In Seconds() -> (seconds since 1Jan1904=w450:timestamp)
        n225 = Bundle By Name(cluster=T19 {"时间标识"=timestamp(0 s since 1904-01-01), "设备"="", "日志信息"="", "流程参数"=""} ("data in"), "时间标识"=w450, "设备"=w444, "日志信息"=w452) -> (w449:T19)
        n226 = call "总磷总氮操作日志.vi"("data in"=w449) -> ()  [unwired: 11 in]
      }
    }
    n227 = case shown="真" w394 {
      tunnel: w397 -> [_ w429]
      tunnel: w398 -> [_ w426]
      frame False {
      }
      frame True {
        n228 = case shown="\"水样测试\"" w429 {
          tunnel: [_ "【水样测试】" ("字符串") "【标样核查】" ("字符串") "【零点核查】" ("字符串") "【跨度核查】" ("字符串") "【空白测试】" ("字符串") "【平行样测试】" ("字符串") "【加标回收】" ("字符串") "【空白校准】" ("字符串") "【标样校准】" ("字符串")] -> w434
          frame "空闲", Default {
          }
          frame "水样测试" {
          }
          frame "标样核查" {
          }
          frame "零点核查" {
          }
          frame "跨度核查" {
          }
          frame "空白测试" {
          }
          frame "平行样测试" {
          }
          frame "加标回收" {
          }
          frame "空白校准" {
          }
          frame "标样校准" {
          }
        }
        n229 = call "id参数转换.vi"("id"=w426) -> ("table输出"=w425:string)  [unwired: 10 in]
        n230 = Concatenate Strings("-->>" ("字符串"), w434, "停止" ("字符串")) -> (w433:string)
        n231 = Get Date/Time In Seconds() -> (seconds since 1Jan1904=w431:timestamp)
        n232 = Bundle By Name(cluster=T19 {"时间标识"=timestamp(0 s since 1904-01-01), "设备"="", "日志信息"="", "流程参数"=""} ("data in"), "时间标识"=w431, "设备"=w425, "日志信息"=w433) -> (w430:T19)
        n233 = call "总磷总氮操作日志.vi"("data in"=w430) -> ()  [unwired: 11 in]
      }
    }
    n234 = call <vilib>:"Boolean Crossing PtByPt.vi"("input"=w419) -> ("crossing"=w401:bool)  [unwired: 2 in]
    n235 = Bundle By Name(cluster=T18 {"启动模式"=enum."跨度核查", "启动参数"=1, "量程"=enum."低量程"} ("参数簇"), "启动参数"=w414, "启动模式"=w416, "量程"=w415) -> (w412:T18)
    n236 = First Call?() -> (First Call?: T/F=w420:bool)
    n237 = Or(x=w401, y=w420) -> (x .or. y?=w418:bool)
    n238 = while {
      tunnel: w418 -> [w544]
      tunnel: w412 -> [w543]
      shift-right: [w538] -> _
      shift-left: _ -> [w540]
      shift-right: [w539] -> _
      shift-left: _ -> [w541]
      shift-right: ["流程路径"] -> _
      shift-left: _ -> [w536]
      stop <- TRUE stop-if-true
      n239 = Not Equal?(x=w536, y="流程路径") -> (x != y?=w534:bool)
      n240 = Or(x=w544, y=w534) -> (x .or. y?=w535:bool)
      n241 = case shown="真" w535 {
        tunnel: [w546 w554] -> w539
        tunnel: [w545 w553] -> w538
        tunnel: w543 -> [_ w548]
        tunnel: w541 -> [w546 _]
        tunnel: w540 -> [w545 _]
        tunnel: "流程路径" -> [_ w547]
        frame False {
        }
        frame True {
          n242 = call "斯坦道XML解析.vi"("添加的路径"=w547, "参数簇"=w548) -> ("步骤时间"=w549:string[], "步骤名"=w551:string[])  [unwired: 8 in]
          n243 = Build Array(w551, w549) -> (w550:string[][])
          n244 = for {
            tunnel: w551 -> [_] mode=indexing
            tunnel: [w555] -> w552 mode=indexing
            i -> [w555]
          }
          n245 = Transpose 2D Array(2D array=w550) -> (transposed array=w553:string[][])
          n246 = Number To Decimal String(number=w552) -> (decimal integer string=w554:string[])  [unwired: 1 in]
        }
      }
      n247 = property on="多列列表框" class="MCListbox (严格)"("ItemNames"=w538, "RowHdrs[]"=w539) -> ()  [unwired: 2 in, 2 out]
    }
    n248 = Not Equal?(x=w408, y=w410) -> (x != y?=w407:bool)
    n249 = case shown="真" w407 {
      frame False {
      }
      frame True {
        n250 = property on="多列列表框" class="MCListbox (严格)"() -> ("ItemNames"=w468:string[][], "Value"=w464:i32)  [unwired: 2 in, 2 out]
        n251 = Index Array(array=w468, index (row)=w464) -> (element=w467:string[])  [unwired: 1 in]
        n252 = Index Array(array=w467) -> (element=w466:string)  [unwired: 1 in]
        n253 = call "过滤筛选流程.vi"("字符串"=w466) -> ("匹配后偏移量"=w465:i32)  [unwired: 10 in]
        n254 = case shown="默认" w465 {
          tunnel: w466 -> [w470 _]
          tunnel: w464 -> [w469 _]
          frame Default {
            n255 = case shown="默认" w470 {
              selector: w470 -> [w476 w483]
              tunnel: [w476 w483] -> w472
              tunnel: [string[] [] ("数组") w478] -> w471
              tunnel: w469 -> [_ w482]
              frame "读数" {
              }
              frame Default {
                n256 = Equal?(x=w482, y=1) -> (x = y?=w480:bool)
                n257 = Select(t=string[] [], s=w480, f="数组") -> (s? t:f=w478:string[])
              }
            }
            n258 = for {
              N: 1 -> [_]
              tunnel: w472 -> [w485]
              shift-right: [w484] -> w473
              shift-left: w471 -> [w486]
              n259 = Search 1D Array(1D array=w486, element=w485) -> (index of element=w489:i32)  [unwired: 1 in]
              n260 = Format Into String(format string="%s" ("格式字符串"), w485) -> (resulting string=w490:string)  [unwired: 2 in, 1 out]
              n261 = Equal?(x=w489, y=-1) -> (x = y?=w487:bool)
              n262 = case shown="真" w487 {
                tunnel: w490 -> [_ w500]
                tunnel: w486 -> [w492 w504]
                tunnel: w485 -> [_ w503]
                tunnel: [w492 w502] -> w484
                frame False {
                }
                frame True {
                  n263 = case shown="\"结束\"" w500 {
                    selector: w500 -> [w527 w530 w533]
                    tunnel: [w527 w529 w532] -> w499
                    frame Default {
                    }
                    frame "初始化" {
                      n264 = Concatenate Strings("-->>" ("字符串"), w530) -> (w529:string)
                    }
                    frame "结束" {
                      n265 = Concatenate Strings("-->>" ("字符串"), w533) -> (w532:string)
                    }
                  }
                  n266 = Insert Into Array(array=w504, new element=w503) -> (w502:string[])  [unwired: 1 in]
                  n267 = global read "VAR总磷总氮全局变量.vi" "状态告警区"() -> (w498:T7)
                  n268 = Unbundle By Name(w498) -> ("工作状态"=w497:T9)
                  n269 = case shown="\"水样测试\"" w497 {
                    tunnel: [_ "【水样测试】" ("字符串") "【标样核查】" ("字符串") "【零点核查】" ("字符串") "【跨度核查】" ("字符串") "【空白测试】" ("字符串") "【平行样测试】" ("字符串") "【加标回收】" ("字符串") "【空白校准】" ("字符串") "【标样校准】" ("字符串")] -> w495
                    frame "空闲", Default {
                    }
                    frame "水样测试" {
                    }
                    frame "标样核查" {
                    }
                    frame "零点核查" {
                    }
                    frame "跨度核查" {
                    }
                    frame "空白测试" {
                    }
                    frame "平行样测试" {
                    }
                    frame "加标回收" {
                    }
                    frame "空白校准" {
                    }
                    frame "标样校准" {
                    }
                  }
                  n270 = global read "VAR总磷总氮全局变量.vi" "状态告警区"() -> (w517:T7)
                  n271 = global read "VAR总磷总氮全局变量.vi" "状态告警区"() -> (w514:T7)
                  n272 = Unbundle By Name(w514) -> ("F0"=w511:sgl, "F1"=w510:sgl, "F2"=w509:sgl, "F3"=w508:sgl, "id"=w507:u16, "flowid"=w506:u16, "量程"=w505:u16)
                  n273 = Unbundle By Name(w517) -> ("id"=w494:u16)
                  n274 = call "id参数转换.vi"("id"=w494) -> ("table输出"=w493:string)  [unwired: 10 in]
                  n275 = Concatenate Strings(w495, w499) -> (w496:string)
                  n276 = Format Into String(format string="F0=%#f,F1=%#f,F2=%#f,F3=%#f,Flow=%d-%-d-%-d" ("格式字符串"), w511, w510, w509, w508, w507, w506, w505) -> (resulting string=w512:string)  [unwired: 2 in, 1 out]
                  n277 = Get Date/Time In Seconds() -> (seconds since 1Jan1904=w515:timestamp)
                  n278 = Bundle By Name(cluster=T19 {"时间标识"=timestamp(0 s since 1904-01-01), "设备"="", "日志信息"="", "流程参数"=""} ("data in"), "时间标识"=w515, "设备"=w493, "日志信息"=w496, "流程参数"=w512) -> (w516:T19)
                  n279 = call "总磷总氮操作日志.vi"("data in"=w516) -> ()  [unwired: 11 in]
                }
              }
            }
            n280 = local write "数组"(w473) -> ()
          }
          frame -1 {
          }
        }
      }
    }
  }
  n281 = flat-sequence {
    tunnel: [w582] -> w6
    frame #0 {
      n282 = call "配置文件路径.vi"() -> ("appended path"=w575:path)  [unwired: 11 in]
      n283 = control-ref of="本VI"() -> (w574:refnum<vi>)
      n284 = call <vilib>:"Open Config Data.vi"("configuration file path"=w575) -> ("error out"=w579:errorcluster, "refnum"=w576:T17)  [unwired: 8 in, 1 out]
      n285 = property class="VI"(reference=w574) -> ("Library.Version"=w573:T21)  [unwired: 1 in, 2 out]
      n286 = vi-ref "总磷总氮断电保存全局变量.vi"() -> (w577:refnum<vi>)
      n287 = Unbundle By Name(w573) -> ("Major"=w571:u16, "Minor"=w570:u16, "Fix"=w569:u16, "Build"=w568:u16)
      n288 = call <userlib>:"Read Panel from INI__ogtk.vi"("error in (no error)"=w579, "VI ref"=w577, "refnum"=w576) -> ("error out"=w580:errorcluster, "refnum out"=w578:T17)  [unwired: 7 in]
      n289 = call <vilib>:"Close Config Data.vi"("error in (no error)"=w580, "refnum"=w578) -> ()  [unwired: 8 in, 2 out]
      n290 = Format Into String(format string="模块版本号：%d.%d.%d.%d" ("格式字符串"), w571, w570, w569, w568) -> (resulting string=→"模块版本号":string)  [unwired: 2 in, 1 out]
    }
    frame #1 {
      n291 = control-ref of="本VI"() -> (w583:refnum<vi>)
      n292 = vi-ref "总磷总氮通讯.vi"() -> (w598:refnum<vi>)
      n293 = global read "总磷总氮断电保存全局变量.vi" "启动参数"() -> (w586:T12)
      n294 = property class="VI"(reference=w583) -> ("Library"=w584:refnum<vi>)  [unwired: 1 in, 2 out]
      n295 = property class="Library"(reference=w584) -> ("LocalName"=w585:string)  [unwired: 1 in, 2 out]
      n296 = Cluster To Array(cluster=w586) -> (array=w587:bool[])
      n297 = vi-ref "总磷总氮测量数据储存.vi"() -> (w606:refnum<vi>)
      n298 = property class="VI"(reference=w598) -> ("Name"=w599:string)  [unwired: 1 in, 2 out]
      n299 = vi-ref "关键参数交互.vi"() -> (w597:refnum<vi>)
      n300 = property on="定时设置" class="定时设置 (严格)"("引用参数"=w585) -> ()  [unwired: 2 in, 2 out]
      n301 = for {
        tunnel: w587 -> [w614] mode=indexing
        tunnel: [w615] -> w589 mode=indexing if=w616
        tunnel: [w615] -> w588 mode=indexing if=w614
        i -> [w615]
        n302 = Not(x=w614) -> (.not. x?=w616:bool)
      }
      n303 = property class="VI"(reference=w606) -> ("Name"=w613:string)  [unwired: 1 in, 2 out]
      n304 = Open VI Reference(type specifier VI Refnum (for type only)=refnum<vi> refnum, vi path=w599, options=128 ("选项")) -> (vi reference=w601:refnum<vi>, error out=w603:errorcluster)  [unwired: 3 in]
      n305 = property class="VI"(reference=w597) -> ("Name"=w591:string)  [unwired: 1 in, 2 out]
      n306 = call-by-ref "开始异步调用"(reference=w601, error in=w603) -> (reference out=w605:refnum<vi>, error out=w604:errorcluster)  [unwired: 12 in]
      n307 = Open VI Reference(type specifier VI Refnum (for type only)=refnum<vi> refnum, vi path=w613, options=128 ("选项")) -> (vi reference=w611:refnum<vi>, error out=w609:errorcluster)  [unwired: 3 in]
      n308 = Close Reference(reference=w605, error in (no error)=w604) -> ()  [unwired: 1 out]
      n309 = Index Array(array=w588) -> (element=w581:i32)  [unwired: 1 in]
      n310 = Open VI Reference(type specifier VI Refnum (for type only)=refnum<vi> refnum, vi path=w591, options=128 ("选项")) -> (vi reference=w593:refnum<vi>, error out=w594:errorcluster)  [unwired: 3 in]
      n311 = property on="参数下拉列表" class="Enum (严格)"("Disabled Items []"=w589, "Val(Sgnl)"=w581) -> ()  [unwired: 2 in, 2 out]
      n312 = call-by-ref "开始异步调用"(reference=w611, error in=w609) -> (reference out=w607:refnum<vi>, error out=w608:errorcluster)  [unwired: 12 in]
      n313 = Close Reference(reference=w607, error in (no error)=w608) -> ()  [unwired: 1 out]
      n314 = call-by-ref "开始异步调用"(reference=w593, error in=w594) -> (reference out=w596:refnum<vi>, error out=w595:errorcluster)  [unwired: 12 in]
      n315 = Close Reference(reference=w596, error in (no error)=w595) -> ()  [unwired: 1 out]
      n316 = call "设置模块队列名.vi"() -> ("Msg"=w582:string)  [unwired: 5 in]
    }
  }
  n317 = Obtain Queue(name (unnamed)=w6, element data type=cluster{"命令":string, "data":variant} {"命令"="", "data"=variant}) -> (queue out=w7:refnum<queue>)  [unwired: 3 in, 2 out]
  n318 = control-ref of="测量模式下拉列表"() -> (w14:refnum<vi>)
  n319 = while {
    tunnel: w7 -> [w621]
    tunnel: [w619] -> _
    stop <- FALSE stop-if-true
    # "定时更新"
    n320 = Get Queue Status(queue=w621) -> (queue out=w618:refnum<queue>, # elements in queue=w617:i32)  [unwired: 2 in, 6 out]
    n321 = Wait (ms)(milliseconds to wait=u32 1000 ("等待时间（毫秒）")) -> ()  [unwired: 1 out]
    n322 = case shown="0" w617 {
      tunnel: w618 -> [_ w629]
      tunnel: [_ w627] -> w619
      frame Default {
      }
      frame 0 {
        n323 = global read "VAR总磷总氮全局变量.vi" "启动队列名称"() -> (w625:cluster{"String":string, "Value":u16}[])
        n324 = Index Array(array=w625) -> (element=w624:cluster{"String":string, "Value":u16})  [unwired: 1 in]
        n325 = Unbundle By Name(w624) -> ("Value"=w623:u16)
        n326 = call "总磷总氮版本号读取.vi"("Slave ID"=w623) -> ("error out"=w627:errorcluster, "固件版本号"=→"固件版本号":string)  [unwired: 9 in]
        n327 = Bundle By Name(cluster=cluster{"命令":string, "data":variant} {"命令"="", "data"=variant} ("元素"), "命令"="读序列号", "data"=w623) -> (w628:cluster{"命令":string, "data":variant})
        n328 = Enqueue Element(queue=w629, element=w628) -> ()  [unwired: 2 in, 3 out]
      }
    }
  }
  n329 = while {
    tunnel: w7 -> [w637]
    stop <- FALSE stop-if-true
    n330 = Get Queue Status(queue=w637) -> (queue out=w635:refnum<queue>, # elements in queue=w634:i32)  [unwired: 2 in, 6 out]
    n331 = Wait (ms)(milliseconds to wait=u32 1000 ("等待时间（毫秒）")) -> ()  [unwired: 1 out]
    n332 = case shown="0" w634 {
      tunnel: w635 -> [_ w653]
      frame Default {
      }
      frame 0 {
        n333 = global read "VAR总磷总氮全局变量.vi" "启动队列名称"() -> (w642:cluster{"String":string, "Value":u16}[])
        n334 = for {
          tunnel: [w671] -> w643 mode=indexing
          tunnel: w642 -> [w672] mode=indexing
          n335 = Unbundle By Name(w672) -> ("Value"=w671:u16)
        }
        n336 = global read "VAR总磷总氮全局变量.vi" "状态告警区"() -> (w645:T7)
        n337 = Unbundle By Name(w645) -> ("系统时间"=w652:timestamp, "工作状态"=w644:T9)
        n338 = for {
          tunnel: w644 -> [w657]
          shift-right: [w658] -> w646
          shift-left: w653 -> [w660]
          tunnel: w643 -> [w654] mode=indexing
          n339 = Equal?(x=w657, y=T9."空闲") -> (x = y?=w655:bool)
          n340 = Bundle By Name(cluster=cluster{"命令":string, "data":variant} {"命令"="", "data"=variant} ("元素"), "命令"="读状态告警区", "data"=w654) -> (w662:cluster{"命令":string, "data":variant})
          n341 = Enqueue Element(queue=w660, element=w662) -> (queue out=w659:refnum<queue>)  [unwired: 2 in, 2 out]
          n342 = case shown="真" w655 {
            tunnel: w659 -> [w664 w667]
            tunnel: w654 -> [_ w666]
            tunnel: [w664 w665] -> w658
            frame False {
            }
            frame True {
              n343 = Bundle By Name(cluster=cluster{"命令":string, "data":variant} {"命令"="", "data"=variant} ("元素"), "命令"="读测量数据区", "data"=w666) -> (w669:cluster{"命令":string, "data":variant})
              n344 = Enqueue Element(queue=w667, element=w669) -> (queue out=w665:refnum<queue>)  [unwired: 2 in, 2 out]
            }
          }
        }
        n345 = Get Date/Time In Seconds() -> (seconds since 1Jan1904=w651:timestamp)
        n346 = Subtract(x=w651, y=w652) -> (x-y=w650:dbl)
        n347 = Absolute Value(x=w650) -> (abs(x)=w649:dbl)
        n348 = Greater Or Equal?(x=w649, y=120.0) -> (x >= y?=w647:bool)
        n349 = case shown="真" w647 {
          tunnel: w646 -> [_ w674]
          frame False {
          }
          frame True {
            n350 = call "总磷总氮启动命令.vi"("参数"=T22 {"站号"=3, "量程切换"=enum."AUTO", "控制命令"=enum."校时", "模式设置"=enum."待机", "测量间隔"=0}) -> ("启动命令"=w673:cluster{"命令":string, "data":variant})  [unwired: 10 in]
            n351 = Enqueue Element(queue=w674, element=w673) -> ()  [unwired: 2 in, 3 out]
          }
        }
      }
    }
    n352 = global read "总磷总氮断电保存全局变量.vi" "流程路径"() -> (w636:path)
    n353 = global read "总磷总氮断电保存全局变量.vi" "MB通信方式选择"() -> (w633:enum16{"串口", "TCP"})
    n354 = local write "流程路径"(w636) -> ()
    n355 = case shown="\"串口\", 默认" w633 {
      tunnel: [w640 w641] -> w632
      frame "串口", Default {
        n356 = global read "总磷总氮断电保存全局变量.vi" "VISA Resource"() -> (w640:refnum<visa-resource-name>)
      }
      frame "TCP" {
        n357 = global read "总磷总氮断电保存全局变量.vi" "IP"() -> (w641:string)
      }
    }
    "字符串 2" <- w632
  }
  n358 = call "设置模块队列名.vi"() -> ("Msg"=w2:string)  [unwired: 5 in]
  n359 = control-ref of="量程参数读取"() -> (w12:refnum<vi>)
  n360 = control-ref of="参数下拉列表"() -> (w15:refnum<vi>)
  n361 = control-ref of="量程下拉列表"() -> (w16:refnum<vi>)
  n362 = control-ref of="公式"() -> (w13:refnum<vi>)
  n363 = Obtain Notifier(name (unnamed)=w2, notification data type=FALSE) -> (notifier out=w1:refnum<notifier>)  [unwired: 2 in, 2 out]
  n364 = while {
    tunnel: w7 -> [w682]
    tunnel: w16 -> [w681]
    tunnel: w15 -> [w680]
    tunnel: w14 -> [w679]
    tunnel: w13 -> [w678]
    tunnel: w12 -> [w677]
    tunnel: w1 -> [w676]
    stop <- FALSE stop-if-true
    n365 = event shown="[4] \"测量模式下拉列表\", \"量程下拉列表\", \"参数下拉列表\": 值改变" {
      selector: _ -> [_ _ _ _ _ _ _ _ _ _ _ _ _ _ _ _ _ _ _ _ _ _ _ _]
      dyn-events: _ -> [_ _ _ _ _ _ _ _ _ _ _ _ _ _ _ _ _ _ _ _ _ _ _ _]
      timeout: _ -> [_ _ _ _ _ _ _ _ _ _ _ _ _ _ _ _ _ _ _ _ _ _ _ _]
      tunnel: w682 -> [_ _ _ _ _ _ w702 w728 _ _ _ _ _ _ w825 _ w834 _ _ _ _ _ _ _]
      tunnel: w681 -> [_ _ _ _ _ _ _ _ _ w748 _ _ _ _ _ _ _ _ _ _ w850 _ _ _]
      tunnel: w680 -> [_ _ _ _ _ _ _ _ _ w752 _ _ _ w803 _ _ _ _ _ _ w848 _ w901 w908]
      tunnel: w679 -> [_ _ _ _ _ _ _ _ _ w750 _ _ _ _ _ _ _ _ _ _ w849 _ _ _]
      tunnel: w678 -> [_ _ _ _ _ _ _ _ _ _ _ _ _ _ _ _ _ _ _ _ w844 _ _ _]
      tunnel: w677 -> [_ _ _ _ _ _ _ _ _ _ _ _ _ _ _ _ _ _ _ _ _ _ w899 _]
      tunnel: [_ _ _ _ w688 _ _ _ _ _ _ _ _ _ _ _ _ _ _ _ _ _ _ _] -> _
      tunnel: w676 -> [_ _ _ _ _ _ _ _ _ _ _ _ _ _ _ _ w830 _ _ _ _ _ _ _]
      event Timeout {
        n366 = event-data() -> ()  [unwired: 1 in, 3 out]
      }
      event "灯值调整": Value Change {
        n367 = event-data() -> ()  [unwired: 1 in, 6 out]
        n368 = call "灯值调整对话框.vi"() -> ()  [unwired: 12 in]
      }
      event "启动参数设置": Value Change {
        n369 = event-data() -> ()  [unwired: 1 in, 6 out]
        n370 = call "启动参数设置.vi"() -> ()  [unwired: 12 in]
      }
      event "布尔": Mouse Down {
        n371 = event-data() -> ("CtlRef"=w685:refnum<vi>)  [unwired: 1 in, 5 out]
        n372 = property class="Bool (严格)"(reference=w685) -> ("Value"=w684:bool)  [unwired: 1 in, 2 out]
        n373 = case shown="真" w684 {
          frame False {
            n374 = call "密码键盘.vi"() -> ("NewNumber"=→"输入密码":dbl)  [unwired: 1 in]
          }
          frame True {
            n375 = local write "输入密码"(u32 0 ("输入密码")) -> ()
          }
        }
      }
      event "测量模式下拉列表", "量程下拉列表", "参数下拉列表": Value Change {
        n376 = event-data() -> ()  [unwired: 1 in, 6 out]
        n377 = local read "测量模式下拉列表"() -> (w691:enum16{"水样测量", "零点核查", "跨度核查", "标样核查", "加标回收"})
        n378 = local read "参数下拉列表"() -> (w690:enum16{"COD", "氨氮", "总氮", "总磷"})
        n379 = local read "量程下拉列表"() -> (w692:enum16{"低量程", "高量程"})
        n380 = Bundle("参数下拉列表"=w690, "测量模式下拉列表"=w691, "量程下拉列表"=w692) -> (w689:T23)  [unwired: 1 in]
        n381 = property on="曲线模型" class="曲线模型 (严格)"("属性"=w689) -> (error out=w688:errorcluster)  [unwired: 2 in, 1 out]
      }
      event "流程固件": Value Change {
        n382 = event-data() -> ()  [unwired: 1 in, 6 out]
        n383 = call "流程固件设置对话框.vi"() -> ()  [unwired: 12 in]
      }
      event "串口设置": Value Change {
        n384 = event-data() -> ()  [unwired: 1 in, 6 out]
        n385 = global read "总磷总氮断电保存全局变量.vi" "MB通信方式选择"() -> (w693:enum16{"串口", "TCP"})
        n386 = global read "总磷总氮断电保存全局变量.vi" "VISA Resource"() -> (w699:refnum<visa-resource-name>)
        n387 = global read "总磷总氮断电保存全局变量.vi" "PORT"() -> (w697:string)
        n388 = global read "总磷总氮断电保存全局变量.vi" "IP"() -> (w698:string)
        n389 = call "串口配置.vi"("PORT"=w697, "IP"=w698, "MB通信方式选择"=w693, "请选择串口:"=w699) -> ("PORT 2"=w695:string, "IP 2"=w696:string, "确认 2"=w700:bool, "VISA资源名称 2"=w701:refnum<visa-resource-name>, "MB通信方式选择 2"=w694:enum16{"串口", "TCP"})  [unwired: 3 in]
        n390 = case shown="真" w700 {
          tunnel: w701 -> [_ w707]
          tunnel: w702 -> [_ w706]
          tunnel: w696 -> [_ w705]
          tunnel: w695 -> [_ w704]
          tunnel: w694 -> [_ w703]
          frame False {
          }
          frame True {
            n391 = flat-sequence {
              tunnel: w707 -> [w712]
              tunnel: w706 -> [w713]
              tunnel: w705 -> [w711]
              tunnel: w704 -> [w710]
              tunnel: w703 -> [w709]
              frame #0 {
                n392 = global write "总磷总氮断电保存全局变量.vi" "IP"(w711) -> ()
                n393 = global write "总磷总氮断电保存全局变量.vi" "PORT"(w710) -> ()
                n394 = global write "总磷总氮断电保存全局变量.vi" "VISA Resource"(w712) -> ()
                n395 = global write "总磷总氮断电保存全局变量.vi" "MB通信方式选择"(w709) -> ()
                n396 = Flush Queue(queue=w713) -> (queue out=w708:refnum<queue>)  [unwired: 1 in, 2 out]
                n397 = Enqueue Element(queue=w708, element=cluster{"命令":string, "data":variant} {"命令"="启用模块", "data"=variant} ("元素")) -> ()  [unwired: 2 in, 3 out]
              }
              frame #1 {
                n398 = call "配置文件路径.vi"() -> ("appended path"=w715:path)  [unwired: 11 in]
                n399 = call <vilib>:"Open Config Data.vi"("configuration file path"=w715) -> ("error out"=w723:errorcluster, "refnum"=w726:T17)  [unwired: 8 in, 1 out]
                n400 = vi-ref "总磷总氮断电保存全局变量.vi"() -> (w725:refnum<vi>)
                n401 = call <userlib>:"Write Panel to INI__ogtk.vi"("error in (no error)"=w723, "VI ref"=w725, "refnum"=w726) -> ("error out"=w722:errorcluster, "refnum out"=w724:T17)  [unwired: 7 in]
                n402 = call <vilib>:"Close Config Data.vi"("error in (no error)"=w722, "refnum"=w724) -> ("error out"=w717:errorcluster, "file path"=w716:path)  [unwired: 8 in]
                n403 = Open/Create/Replace File(file path (use dialog)=w716, error in=w717) -> (refnum out=w720:refnum<file>, error out=w721:errorcluster)  [unwired: 4 in, 1 out]
                n404 = Flush File(refnum=w720, error in=w721) -> (refnum out=w719:refnum<file>, error out=w718:errorcluster)
                n405 = Close File(refnum=w719, error in=w718) -> ()  [unwired: 2 out]
              }
            }
          }
        }
      }
      event "模块启用": Value Change {
        n406 = event-data() -> ("OldVal"=w729:bool)  [unwired: 1 in, 5 out]
        n407 = Flush Queue(queue=w728) -> (queue out=w727:refnum<queue>)  [unwired: 1 in, 2 out]
        n408 = case shown="假" w729 {
          tunnel: w727 -> [w730 w732]
          frame False {
            n409 = Enqueue Element(queue=w730, element=cluster{"命令":string, "data":variant} {"命令"="停用模块", "data"=variant} ("元素")) -> ()  [unwired: 2 in, 3 out]
          }
          frame True {
            n410 = Enqueue Element(queue=w732, element=cluster{"命令":string, "data":variant} {"命令"="启用模块", "data"=variant} ("元素")) -> ()  [unwired: 2 in, 3 out]
          }
        }
      }
      event "流程路径": Value Change {
        n411 = event-data() -> ()  [unwired: 1 in, 6 out]
        n412 = flat-sequence {
          frame #0 {
            n413 = local read "流程路径"() -> (w734:path)
            n414 = global write "总磷总氮断电保存全局变量.vi" "流程路径"(w734) -> ()
          }
          frame #1 {
            n415 = call "配置文件路径.vi"() -> ("appended path"=w735:path)  [unwired: 11 in]
            n416 = call <vilib>:"Open Config Data.vi"("configuration file path"=w735) -> ("error out"=w743:errorcluster, "refnum"=w746:T17)  [unwired: 8 in, 1 out]
            n417 = vi-ref "总磷总氮断电保存全局变量.vi"() -> (w745:refnum<vi>)
            n418 = call <userlib>:"Write Panel to INI__ogtk.vi"("error in (no error)"=w743, "VI ref"=w745, "refnum"=w746) -> ("error out"=w742:errorcluster, "refnum out"=w744:T17)  [unwired: 7 in]
            n419 = call <vilib>:"Close Config Data.vi"("error in (no error)"=w742, "refnum"=w744) -> ("error out"=w737:errorcluster, "file path"=w736:path)  [unwired: 8 in]
            n420 = Open/Create/Replace File(file path (use dialog)=w736, error in=w737) -> (refnum out=w740:refnum<file>, error out=w741:errorcluster)  [unwired: 4 in, 1 out]
            n421 = Flush File(refnum=w740, error in=w741) -> (refnum out=w739:refnum<file>, error out=w738:errorcluster)
            n422 = Close File(refnum=w739, error in=w738) -> ()  [unwired: 2 out]
          }
        }
      }
      event "公式一键写入": Value Change {
        n423 = event-data() -> ()  [unwired: 1 in, 6 out]
        n424 = property class="Enum (严格)"(reference=w752) -> ("Value"=w751:enum16{"COD", "氨氮", "总氮", "总磷"})  [unwired: 1 in, 2 out]
        n425 = property class="Enum (严格)"(reference=w750) -> ("Value"=w749:enum16{"水样测量", "零点核查", "跨度核查", "标样核查", "加标回收"})  [unwired: 1 in, 2 out]
        n426 = property class="Enum (严格)"(reference=w748) -> ("Value"=w747:enum16{"低量程", "高量程"})  [unwired: 1 in, 2 out]
        n427 = local read "公式"() -> (w754:cluster{"X^2":dbl, "X":dbl, "b":dbl})
        n428 = call "公式复合写入.vi"("公式"=w754, "量程下拉列表"=w747, "测量模式下拉列表"=w749, "参数下拉列表"=w751) -> ("模型复制"=w753:T24)  [unwired: 7 in]
        n429 = invoke on="曲线模型" class="曲线模型 (严格)" method="模型复制.vi"("模型复制"=w753) -> ()  [unwired: 3 in, 4 out]
      }
      event "曲线模型": Value Change {
        n430 = event-data() -> ()  [unwired: 1 in, 6 out]
        n431 = Unbundle By Name("曲线模型") -> ("X^2"=w758:dbl, "X"=w757:dbl, "B"=w756:dbl)
        n432 = Bundle("X^2"=w758, "X"=w757, "B"=w756) -> (w755:cluster{"X^2":dbl, "X":dbl, "B":dbl})  [unwired: 1 in]
        n433 = local write "公式"(w755) -> ()
      }
      event "质控参数设置": Value Change {
        n434 = event-data() -> ()  [unwired: 1 in, 6 out]
        n435 = global read "总磷总氮断电保存全局变量.vi" "质控参数设置"() -> (w762:T25)
        n436 = call "总磷总氮质控参数设置.vi"("质控参数设置"=w762) -> ("质控参数设置 2"=w760:T25, "check？"=w761:bool)  [unwired: 9 in]
        n437 = case shown="真" w761 {
          tunnel: w762 -> [_ w764]
          tunnel: w760 -> [_ w763]
          frame False {
          }
          frame True {
            n438 = flat-sequence {
              tunnel: w764 -> [_]
              tunnel: w763 -> [w765]
              frame #0 {
                n439 = global write "总磷总氮断电保存全局变量.vi" "质控参数设置"(w765) -> ()
              }
              frame #1 {
                n440 = call "配置文件路径.vi"() -> ("appended path"=w766:path)  [unwired: 11 in]
                n441 = call <vilib>:"Open Config Data.vi"("configuration file path"=w766) -> ("error out"=w774:errorcluster, "refnum"=w777:T17)  [unwired: 8 in, 1 out]
                n442 = vi-ref "总磷总氮断电保存全局变量.vi"() -> (w776:refnum<vi>)
                n443 = call <userlib>:"Write Panel to INI__ogtk.vi"("error in (no error)"=w774, "VI ref"=w776, "refnum"=w777) -> ("error out"=w773:errorcluster, "refnum out"=w775:T17)  [unwired: 7 in]
                n444 = call <vilib>:"Close Config Data.vi"("error in (no error)"=w773, "refnum"=w775) -> ("error out"=w768:errorcluster, "file path"=w767:path)  [unwired: 8 in]
                n445 = Open/Create/Replace File(file path (use dialog)=w767, error in=w768) -> (refnum out=w771:refnum<file>, error out=w772:errorcluster)  [unwired: 4 in, 1 out]
                n446 = Flush File(refnum=w771, error in=w772) -> (refnum out=w770:refnum<file>, error out=w769:errorcluster)
                n447 = Close File(refnum=w770, error in=w769) -> ()  [unwired: 2 out]
              }
            }
          }
        }
      }
      event "仪器参数": Value Change {
        n448 = event-data() -> ()  [unwired: 1 in, 6 out]
        n449 = global read "总磷总氮断电保存全局变量.vi" "COD仪器参数"() -> (w783:T26)
        n450 = global read "总磷总氮断电保存全局变量.vi" "氨氮仪器参数"() -> (w782:T26)
        n451 = global read "总磷总氮断电保存全局变量.vi" "总氮仪器参数"() -> (w781:T26)
        n452 = global read "总磷总氮断电保存全局变量.vi" "总磷仪器参数"() -> (w780:T26)
        n453 = Bundle("COD仪器参数"=w783, "氨氮仪器参数"=w782, "总氮仪器参数"=w781, "总磷仪器参数"=w780) -> (w779:T27)  [unwired: 1 in]
        n454 = call "仪器参数设置.vi"("仪器参数"=w779) -> ("仪器参数 2"=w778:T27, "check？"=w784:bool)  [unwired: 9 in]
        n455 = case shown="真" w784 {
          tunnel: w778 -> [_ w785]
          frame False {
          }
          frame True {
            n456 = flat-sequence {
              tunnel: w785 -> [w790]
              frame #0 {
                n457 = Unbundle By Name(w790) -> ("COD仪器参数"=w788:T26, "氨氮仪器参数"=w787:T26, "总氮仪器参数"=w789:T26, "总磷仪器参数"=w786:T26)
                n458 = global write "总磷总氮断电保存全局变量.vi" "COD仪器参数"(w788) -> ()
                n459 = global write "总磷总氮断电保存全局变量.vi" "氨氮仪器参数"(w787) -> ()
                n460 = global write "总磷总氮断电保存全局变量.vi" "总氮仪器参数"(w789) -> ()
                n461 = global write "总磷总氮断电保存全局变量.vi" "总磷仪器参数"(w786) -> ()
              }
              frame #1 {
                n462 = call "配置文件路径.vi"() -> ("appended path"=w791:path)  [unwired: 11 in]
                n463 = call <vilib>:"Open Config Data.vi"("configuration file path"=w791) -> ("error out"=w799:errorcluster, "refnum"=w802:T17)  [unwired: 8 in, 1 out]
                n464 = vi-ref "总磷总氮断电保存全局变量.vi"() -> (w801:refnum<vi>)
                n465 = call <userlib>:"Write Panel to INI__ogtk.vi"("error in (no error)"=w799, "VI ref"=w801, "refnum"=w802) -> ("error out"=w798:errorcluster, "refnum out"=w800:T17)  [unwired: 7 in]
                n466 = call <vilib>:"Close Config Data.vi"("error in (no error)"=w798, "refnum"=w800) -> ("error out"=w793:errorcluster, "file path"=w792:path)  [unwired: 8 in]
                n467 = Open/Create/Replace File(file path (use dialog)=w792, error in=w793) -> (refnum out=w796:refnum<file>, error out=w797:errorcluster)  [unwired: 4 in, 1 out]
                n468 = Flush File(refnum=w796, error in=w797) -> (refnum out=w795:refnum<file>, error out=w794:errorcluster)
                n469 = Close File(refnum=w795, error in=w794) -> ()  [unwired: 2 out]
              }
            }
          }
        }
      }
      event "测试量程配置": Value Change {
        n470 = event-data() -> ()  [unwired: 1 in, 6 out]
        n471 = flat-sequence {
          tunnel: w803 -> [w806]
          frame #0 {
            n472 = property class="Enum (严格)"(reference=w806) -> ("Value"=w805:enum16{"COD", "氨氮", "总氮", "总磷"})  [unwired: 1 in, 2 out]
            n473 = case shown="默认" w805 {
              tunnel: "测试量程配置" -> [_ w807 w808 w809 w810]
              frame Default {
              }
              frame "COD" {
                n474 = global write "总磷总氮断电保存全局变量.vi" "COD自动测试量程配置"(w807) -> ()
              }
              frame "氨氮" {
                n475 = global write "总磷总氮断电保存全局变量.vi" "氨氮自动测试量程配置"(w808) -> ()
              }
              frame "总氮" {
                n476 = global write "总磷总氮断电保存全局变量.vi" "总氮自动测试量程配置"(w809) -> ()
              }
              frame "总磷" {
                n477 = global write "总磷总氮断电保存全局变量.vi" "总磷自动测试量程配置"(w810) -> ()
              }
            }
          }
          frame #1 {
            n478 = call "配置文件路径.vi"() -> ("appended path"=w811:path)  [unwired: 11 in]
            n479 = call <vilib>:"Open Config Data.vi"("configuration file path"=w811) -> ("error out"=w819:errorcluster, "refnum"=w822:T17)  [unwired: 8 in, 1 out]
            n480 = vi-ref "总磷总氮断电保存全局变量.vi"() -> (w821:refnum<vi>)
            n481 = call <userlib>:"Write Panel to INI__ogtk.vi"("error in (no error)"=w819, "VI ref"=w821, "refnum"=w822) -> ("error out"=w818:errorcluster, "refnum out"=w820:T17)  [unwired: 7 in]
            n482 = call <vilib>:"Close Config Data.vi"("error in (no error)"=w818, "refnum"=w820) -> ("error out"=w813:errorcluster, "file path"=w812:path)  [unwired: 8 in]
            n483 = Open/Create/Replace File(file path (use dialog)=w812, error in=w813) -> (refnum out=w816:refnum<file>, error out=w817:errorcluster)  [unwired: 4 in, 1 out]
            n484 = Flush File(refnum=w816, error in=w817) -> (refnum out=w815:refnum<file>, error out=w814:errorcluster)
            n485 = Close File(refnum=w815, error in=w814) -> ()  [unwired: 2 out]
          }
        }
      }
      event "手动启动": Value Change {
        n486 = event-data() -> ()  [unwired: 1 in, 6 out]
        n487 = call "总磷总氮启动参数对话框.vi"() -> ("确认"=w823:bool, "元素"=w824:cluster{"命令":string, "data":variant})  [unwired: 10 in]
        n488 = case shown="真" w823 {
          tunnel: w825 -> [_ w828]
          tunnel: w824 -> [_ w827]
          frame False {
          }
          frame True {
            n489 = Flush Queue(queue=w828) -> (queue out=w826:refnum<queue>)  [unwired: 1 in, 2 out]
            n490 = Enqueue Element(queue=w826, element=w827) -> ()  [unwired: 2 in, 3 out]
          }
        }
      }
      event "单步测试": Value Change {
        n491 = event-data() -> ()  [unwired: 1 in, 6 out]
        n492 = call "总磷单步调试对话框.vi"() -> ()  [unwired: 12 in]
      }
      event "停止": Value Change {
        n493 = event-data() -> ()  [unwired: 1 in, 6 out]
        n494 = Send Notification(notification=TRUE ("通知"), notifier=w830) -> ()  [unwired: 1 in, 2 out]
        n495 = Enqueue Element(queue=w834, element=cluster{"命令":string, "data":variant} {"命令"="启动", "data"=variant(cluster{"站号":u16, "控制命令输出":u16[]} {"站号"=1, "控制命令输出"=[2816]})} ("元素")) -> (queue out=w831:refnum<queue>)  [unwired: 2 in, 2 out]
        n496 = Enqueue Element(queue=w831, element=cluster{"命令":string, "data":variant} {"命令"="启动", "data"=variant(cluster{"站号":u16, "控制命令输出":u16[]} {"站号"=2, "控制命令输出"=[2816]})} ("元素")) -> ()  [unwired: 2 in, 3 out]
      }
      event "参数设置": Value Change {
        n497 = event-data() -> ()  [unwired: 1 in, 6 out]
        n498 = property on="窗格" class="Pane"("Origin"=T13 {"Horizontal"=0, "Vertical"=628} ("原点")) -> ()  [unwired: 2 in, 2 out]
      }
      event "返回": Value Change {
        n499 = event-data() -> ()  [unwired: 1 in, 6 out]
        n500 = property on="窗格" class="Pane"("Origin"=T13 {"Horizontal"=0, "Vertical"=0} ("原点")) -> ()  [unwired: 2 in, 2 out]
      }
      event "公式.X^2", "公式.X", "公式.b", "量程参数读取.测量精度", "量程参数读取.检出限", "量程参数读取.上限", "量程参数读取.下限", "量程参数读取.阈值（低->高）", "量程参数读取.阈值（高->低）", "量程参数读取.稀释度": Mouse Down {
        n501 = event-data() -> ("CtlRef"=w840:refnum<vi>)  [unwired: 1 in, 7 out]
        n502 = property class="DigNum (严格)"(reference=w840) -> (reference out=w838:refnum<vi>, "Value"=w839:dbl)  [unwired: 1 in, 1 out]
        n503 = call "数字键盘.vi"("OldNumber"=w839) -> ("NewNumber"=w837:dbl)
        n504 = property class="DigNum (严格)"(reference=w838, "Val(Sgnl)"=w837) -> ()  [unwired: 1 in, 2 out]
      }
      event "读公式": Value Change {
        n505 = event-data() -> ()  [unwired: 1 in, 6 out]
        n506 = property class="Enum (严格)"(reference=w848) -> ("Value"=w847:enum16{"COD", "氨氮", "总氮", "总磷"})  [unwired: 1 in, 2 out]
        n507 = property class="Enum (严格)"(reference=w849) -> ("Value"=w846:enum16{"水样测量", "零点核查", "跨度核查", "标样核查", "加标回收"})  [unwired: 1 in, 2 out]
        n508 = property class="Enum (严格)"(reference=w850) -> ("Value"=w845:enum16{"低量程", "高量程"})  [unwired: 1 in, 2 out]
        n509 = call "总磷总氮公式读取.vi"("量程"=w845, "测量模式"=w846, "测量参数"=w847) -> ("error out"=w842:errorcluster, "公式"=w843:cluster{"X^2":dbl, "X":dbl, "b":dbl})  [unwired: 7 in]
        n510 = property class="Clust (严格)"(reference=w844, "Value"=w843) -> ()  [unwired: 1 in, 2 out]
        n511 = case shown="错误" w842 {
          tunnel: ["读取成功" ("消息") "读取失败" ("消息")] -> w841
          frame No Error {
          }
          frame Error {
          }
        }
        n512 = One Button Dialog(message=w841) -> ()  [unwired: 1 in, 1 out]
      }
      event "写公式": Value Change {
        n513 = event-data() -> ()  [unwired: 1 in, 6 out]
        n514 = call "总磷总氮公式写入.vi"("公式"="公式", "量程"="量程下拉列表", "测量模式"="测量模式下拉列表", "测量参数"="参数下拉列表") -> ("error out"=w857:errorcluster)  [unwired: 7 in]
        n515 = case shown="无错误" w857 {
          tunnel: ["写入成功" ("消息") "写入失败" ("消息")] -> w858
          tunnel: "测量模式下拉列表" -> [w867 _]
          tunnel: "量程下拉列表" -> [w865 _]
          tunnel: "参数下拉列表" -> [w860 _]
          tunnel: "公式" -> [w859 _]
          frame No Error {
            n516 = Equal?(x=w867, y=enum16{"水样测量", "零点核查", "跨度核查", "标样核查", "加标回收"}."水样测量" ("测量模式下拉列表")) -> (x = y?=w863:bool)
            n517 = Equal?(x=w865, y=enum16{"低量程", "高量程"}."低量程" ("量程下拉列表")) -> (x = y?=w862:bool)
            n518 = And(x=w863, y=w862) -> (x .and. y?=w861:bool)
            n519 = case shown="真" w861 {
              tunnel: w860 -> [_ w870]
              tunnel: w859 -> [_ w869]
              frame False {
              }
              frame True {
                n520 = case shown="\"COD\"" w870 {
                  tunnel: w869 -> [w871 w877 w883 w889]
                  frame "总磷", Default {
                    n521 = Unbundle By Name(w871) -> ("X^2"=w874:dbl, "X"=w873:dbl, "b"=w872:dbl)
                    n522 = global read "总磷总氮断电保存全局变量.vi" "总磷仪器参数"() -> (w875:T26)
                    n523 = Bundle By Name(cluster=w875, "曲线截距"=w872, "曲线斜率"=w873, "二次多项式系数"=w874) -> (w876:T26)
                    n524 = global write "总磷总氮断电保存全局变量.vi" "总磷仪器参数"(w876) -> ()
                  }
                  frame "总氮" {
                    n525 = Unbundle By Name(w877) -> ("X^2"=w880:dbl, "X"=w879:dbl, "b"=w878:dbl)
                    n526 = global read "总磷总氮断电保存全局变量.vi" "总氮仪器参数"() -> (w881:T26)
                    n527 = Bundle By Name(cluster=w881, "曲线截距"=w878, "曲线斜率"=w879, "二次多项式系数"=w880) -> (w882:T26)
                    n528 = global write "总磷总氮断电保存全局变量.vi" "总氮仪器参数"(w882) -> ()
                  }
                  frame "COD" {
                    n529 = Unbundle By Name(w883) -> ("X^2"=w886:dbl, "X"=w885:dbl, "b"=w884:dbl)
                    n530 = global read "总磷总氮断电保存全局变量.vi" "COD仪器参数"() -> (w887:T26)
                    n531 = Bundle By Name(cluster=w887, "曲线截距"=w884, "曲线斜率"=w885, "二次多项式系数"=w886) -> (w888:T26)
                    n532 = global write "总磷总氮断电保存全局变量.vi" "COD仪器参数"(w888) -> ()
                  }
                  frame "氨氮" {
                    n533 = Unbundle By Name(w889) -> ("X^2"=w892:dbl, "X"=w891:dbl, "b"=w890:dbl)
                    n534 = global read "总磷总氮断电保存全局变量.vi" "氨氮仪器参数"() -> (w893:T26)
                    n535 = Bundle By Name(cluster=w893, "曲线截距"=w890, "曲线斜率"=w891, "二次多项式系数"=w892) -> (w894:T26)
                    n536 = global write "总磷总氮断电保存全局变量.vi" "氨氮仪器参数"(w894) -> ()
                  }
                }
              }
            }
          }
          frame Error {
          }
        }
        n537 = One Button Dialog(message=w858) -> ()  [unwired: 1 in, 1 out]
      }
      event "量程切换阈值读取": Value Change {
        n538 = event-data() -> ()  [unwired: 1 in, 6 out]
        n539 = property class="Enum (严格)"(reference=w901) -> ("Value"=w900:enum16{"COD", "氨氮", "总氮", "总磷"})  [unwired: 1 in, 2 out]
        n540 = call "总磷总氮量程读取.vi"("测量参数"=w900) -> ("error out"=w897:errorcluster, "量程参数读取"=w896:T28)  [unwired: 9 in]
        n541 = property class="Clust (严格)"(reference=w899, "Value"=w896) -> ()  [unwired: 1 in, 2 out]
        n542 = case shown="错误" w897 {
          tunnel: ["读取成功" ("消息") "读取失败" ("消息")] -> w898
          frame No Error {
          }
          frame Error {
          }
        }
        n543 = One Button Dialog(message=w898) -> ()  [unwired: 1 in, 1 out]
      }
      event "量程切换阈值写入": Value Change {
        n544 = event-data() -> ()  [unwired: 1 in, 6 out]
        n545 = property class="Enum (严格)"(reference=w908) -> ("Value"=w904:enum16{"COD", "氨氮", "总氮", "总磷"})  [unwired: 1 in, 2 out]
        n546 = call "总磷总氮量程写入.vi"("量程参数写入"="量程参数读取", "测量参数"=w904) -> ("error out"=w906:errorcluster)  [unwired: 8 in]
        n547 = case shown="无错误" w906 {
          tunnel: ["写入成功" ("消息") "写入失败" ("消息")] -> w907
          frame No Error {
          }
          frame Error {
          }
        }
        n548 = One Button Dialog(message=w907) -> ()  [unwired: 1 in, 1 out]
      }
    }
  }
